vi "Autonomous Independent.vi"() -> ()   [LabVIEW 2016]
doc: "This VI is called when autonomous begins, and will automatically be terminated when autonomous ends. You can carry out timed or sensor driven robot movement independently without needing to return to the caller."
uses:
  <vilib>/Rock Robotics/WPI/ThirdParty/CanMotor/TalonSRX/WPI_CANTalonSRX_APIFeedbackSelect.ctl
  <vilib>/Rock Robotics/WPI/ThirdParty/CanMotor/TalonSRX/WPI_CANTalonSRX_Params.ctl
  <vilib>/Rock Robotics/WPI/ThirdParty/CanMotor/TalonSRX/WPI_CANTalonSRX_APIControlMode.ctl
  <vilib>/Rock Robotics/WPI/Utilities/WPI_GetSetVariantRefNum.vi
  <vilib>/Rock Robotics/Network Tables/NT Read String.vi
  <vilib>/Rock Robotics/Network Tables/NT Write Numeric Array.vi
  <vilib>/Rock Robotics/WPI/RobotDrive/WPI_RobotDriveArcadeDrive_Standard(NoSaturation).vi
  Robot Global Data.vi
panel:
  out "Distance":dbl
  out "Current":dbl
  out "CURRENT":dbl
  out "Distance 5":dbl
  out "Distance 4":dbl
  out "Distance 3":dbl
  out "RIGHT SIDE":dbl
  out "Encoder Position 4":dbl
  out "Encoder Position 3":dbl
  out "Encoder Position":dbl
  out "Encoder Position 2":dbl
  # "Be sure to right-click and choose Data Operations>>Make Current Value default if you want to save the array values with the VI"
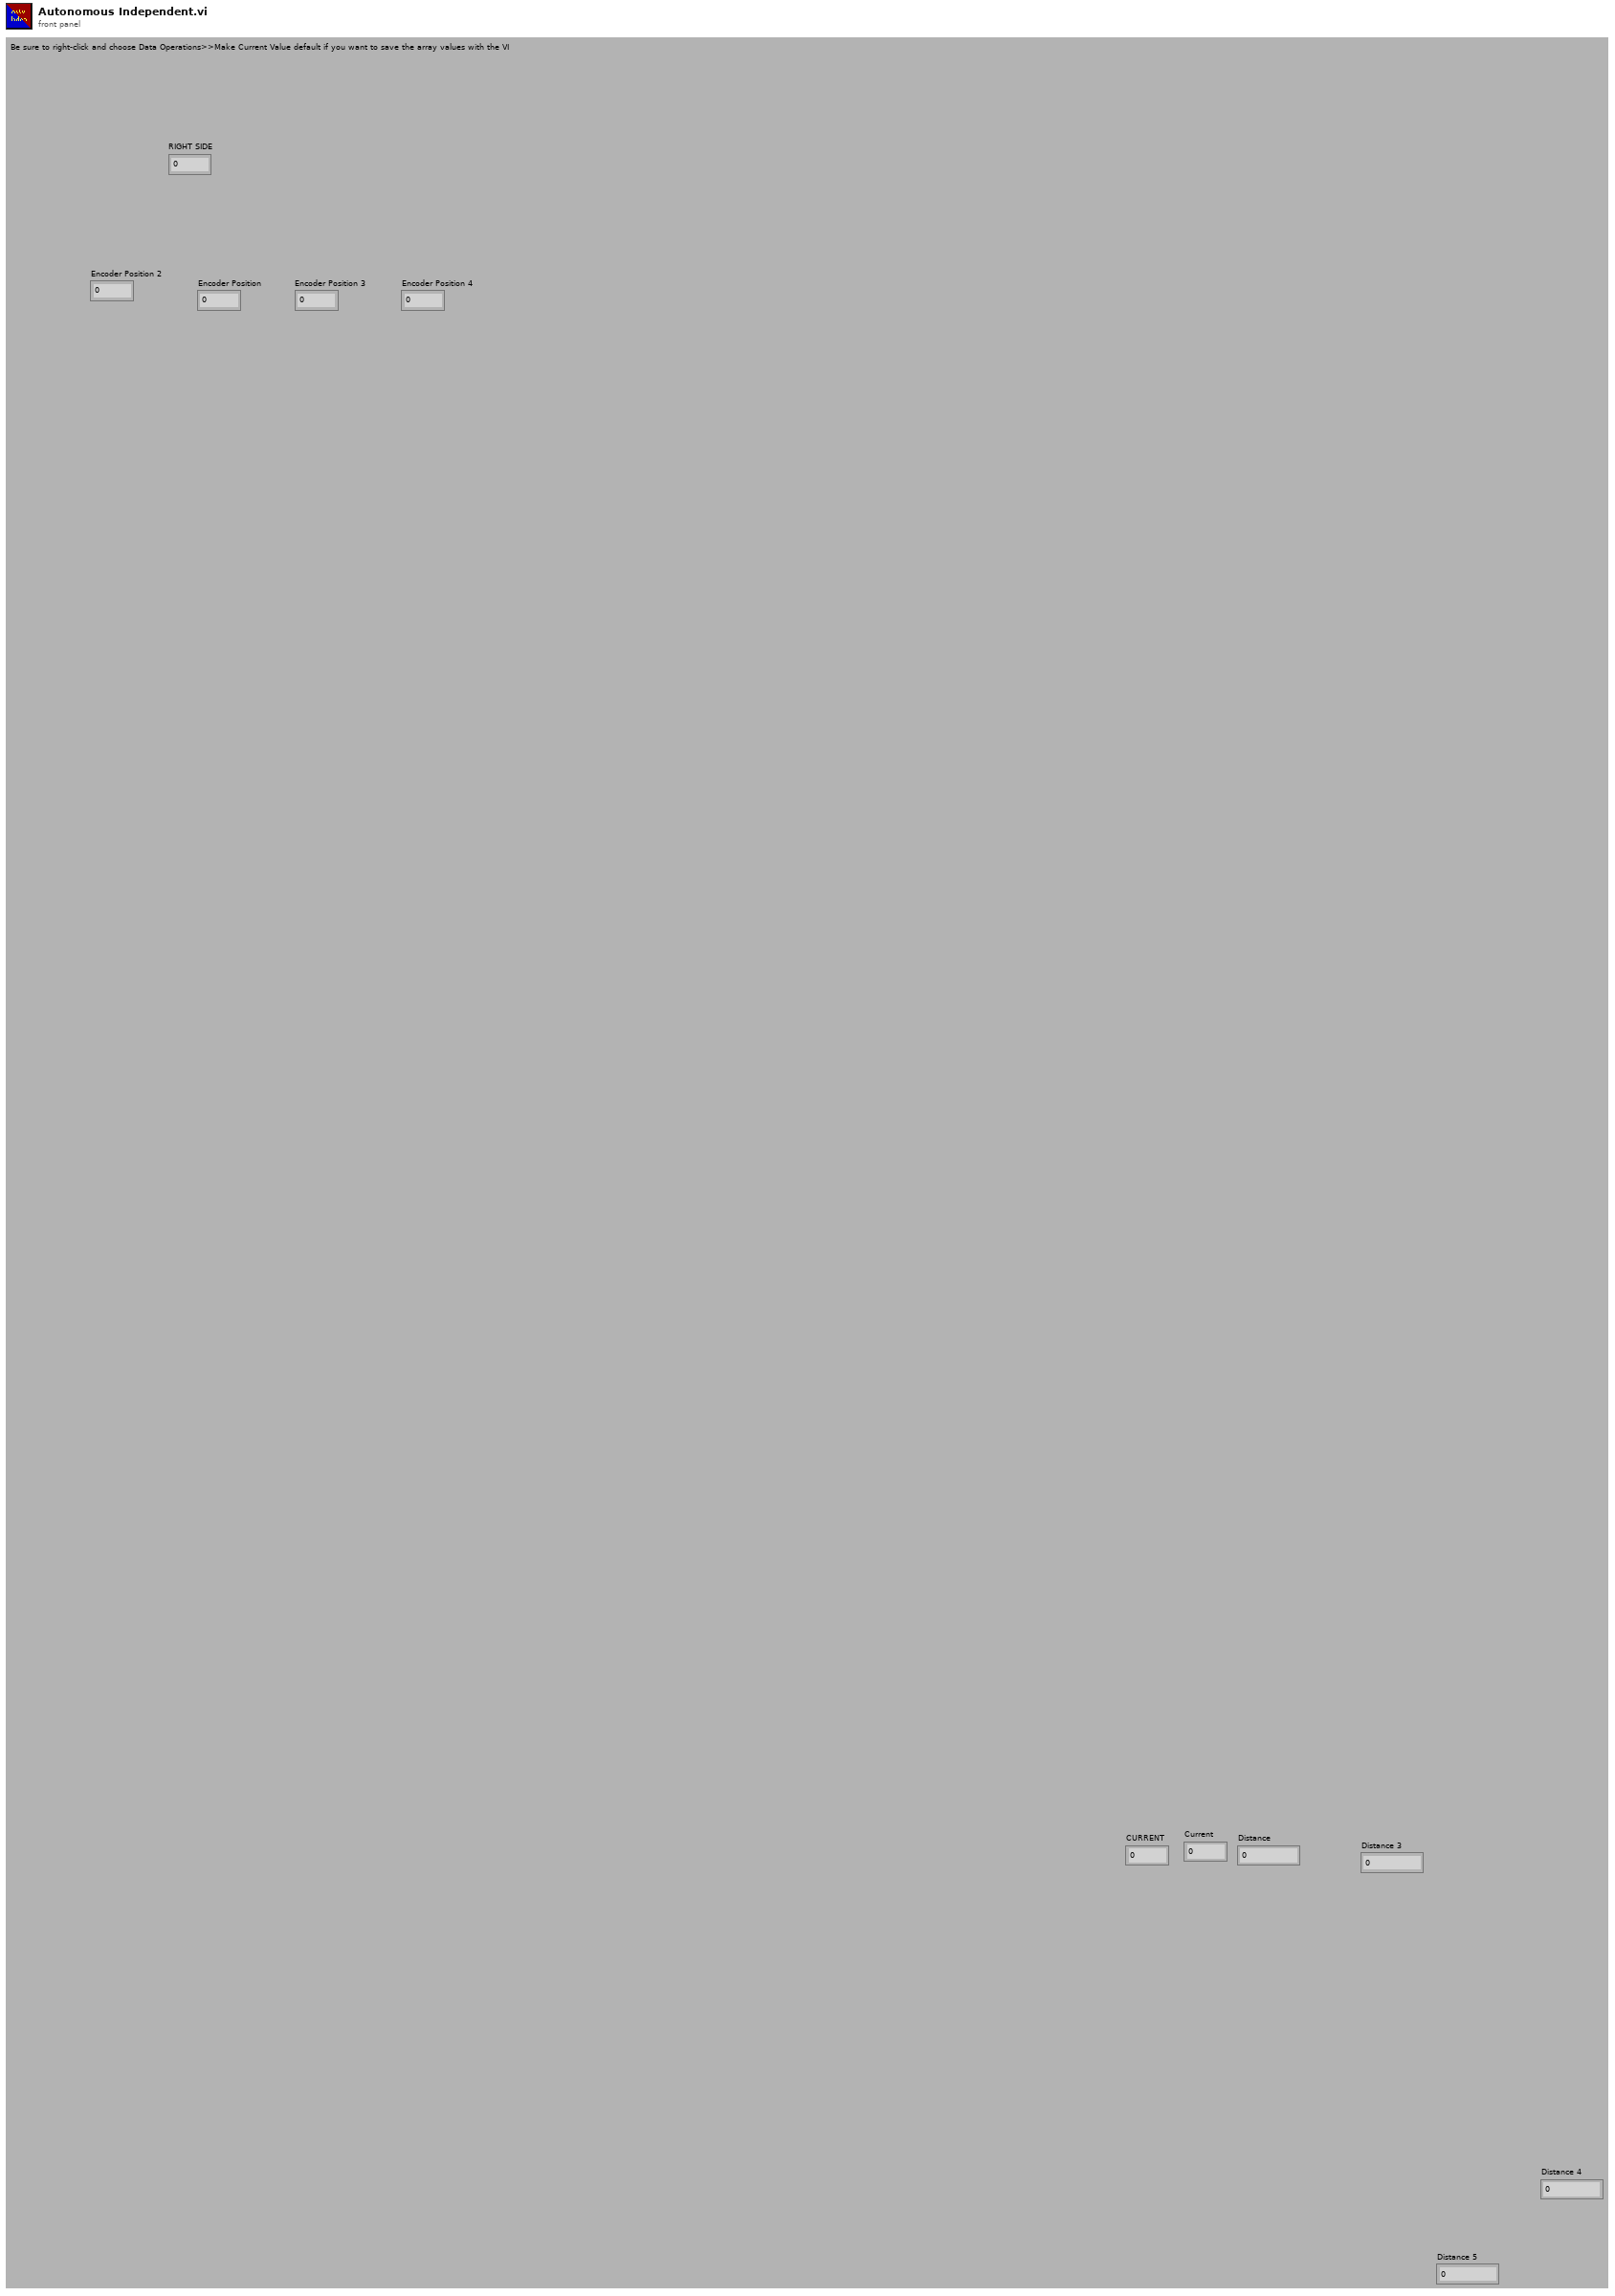
[diagram p1: front panel]
types:
  T1 = typedef "WPI_JoystickDevRef.ctl" = cluster{"Device":T2}
  T2 = typedef "WPI_JoystickDeviceEnum.ctl" = enum16{"USB 0", "USB 1", "USB 2", "USB 3", "USB 4", "USB 5"}
  T3 = typedef "WPI_EncoderDevRef.ctl" = cluster{"DevStatus":errorcluster, "EncoderIndex":T4, "CounterIndex":T5, "DistancePerCount":dbl, "Decoding Type":T6}
  T4 = typedef "FPGA_EncoderIdx.ctl" = enum8{"Enc 0", "Enc 1", "Enc 2", "Enc 3", "Enc 4", "Enc 5", "Enc 6", "Enc 7", "Invalid"}
  T5 = typedef "FPGA_CounterCtrSystemIndex.ctl" = enum8{"Ctr 0", "Ctr 1", "Ctr 2", "Ctr 3", "Ctr 4", "Ctr 5", "Ctr 6", "Ctr 7", "Invalid"}
  T6 = typedef "WPI_EncoderType.ctl" = enum16{"1x", "2x", "4x"}
  T7 = typedef "WPI_MotorControlDeviceRef.ctl" = cluster{"DeviceStatus":errorcluster, "Type":T8, "PWM":cluster{"PWM Channel":T9, "DeadBand":T10}, "CAN":cluster{"Device Number":u8, "SetOutput VI Ref":variant, "GetOutput VI Ref":variant, "Enable VI Ref":variant, "Disable VI Ref":variant, "Data":variant}, "Invert":bool}
  T8 = typedef "WPI_MotorControlType.ctl" = enum16{"PWM", "CAN"}
  T9 = typedef "FPGA_DIOPWMChannel.ctl" = enum8{"PWM 0", "PWM 1", "PWM 2", "PWM 3", "PWM 4", "PWM 5", "PWM 6", "PWM 7", "PWM 8", "PWM 9", "PWM MXP 0", "PWM MXP 1", "PWM MXP 2", "PWM MXP 3", "PWM MXP 4", "PWM MXP 5", "PWM MXP 6", "PWM MXP 7", "PWM MXP 8", "PWM MXP 9", "Invalid"}
  T10 = typedef "WPI_PWMDeadband.ctl" = cluster{"Name":string, "maxPositivePwm":i32, "minPositivePwm":i32, "centerPwm":i32, "maxNegativePwm":i32, "minNegativePwm":i32, "angularRange":u16}
  T11 = typedef "WPI_RobotDriveDevRef.ctl" = cluster{"DevStatus":errorcluster, "Motors[]":T7[], "Square Inputs":bool, "Max Output":dbl}
  T12 = typedef "WPI_CANTalonSRX_APIFeedbackSelect.ctl" = enum16{"Digital Quadrature Encoder", "Analog Potentiometer", "Analog Encoder", "Count on Quad-A (Rising-Edge)", "Count on Quad-A (Falling-Edge)", "CTR Magnetic Enc (Absolute)", "CTR Magnetic Enc (Relative)", "Pulse Width"}
  T13 = typedef "WPI_CANTalonSRX_APIControlMode.ctl" = enum8{"Percent VBus", "Speed", "Position", "Slave", "Unchanged / Invalid", "Voltage Compensation", "Current", "Motion Profile", "Motion Magic"}
  T14 = typedef "WPI_CANTalonSRX_Params.ctl" = u8
  T15 = typedef "WPI_CANTalonSRX_GlobalStatus.ctl" = cluster{"Applied Throttle":dbl, "Module Enabled":bool, "CAN Error":errorcluster, "Closed Loop Error":dbl, "Forward Limit Switch Closed":bool, "Reverse Limit Switch Closed":bool, "Sensor Position":dbl, "Sensor Velocity":dbl, "Current":dbl, "Sticky Fault - Over Temp":bool, "Sticky Fault - Under Voltage":bool, "Sticky Fault - Forward Limit":bool, "Sticky Fault - Reverse Limit":bool, "Sticky Fault - Forward Soft Limit":bool, "Sticky Fault - Reverse Soft Limit":bool, "Brake is Enabled":bool, "Encoder Position":dbl, "Encoder Velocity":dbl, "Encoder Index Count":dbl, "Encoder A Pin State":bool, "Encoder B Pin State":bool, "Encoder Index Pin State":bool, "Analog In":dbl, "Analog In Velocity":dbl, "Temperature (C)":dbl, "Battery Voltage":dbl, "Control 5 Is Supported":bool, "Current Profile Slot Select":dbl, "Pos Div 8":bool, "Vel Div 4":bool, "Pulse Width Position":i32, "Pulse Width Velocity":i32, "Pulse Width Rise To Rise (us)":i32, "Pulse Width Rise To Fall (us)":i32, "Mot Prof Active Is Under Run":bool, "Mot Prof Active Has Under Run":bool, "Mot Prof Active Is Last":bool, "Mot Prof Active Velocity Only":bool, "Mot Prof Active Is Valid":bool, "Mot Prof Buffer Is Full":bool, "Mot Prof Active Profile Slot Select":i32, "Mot Prof NextID":i32, "Mot Prof Count":i32, "Mot Prof Active Velocity":dbl, "Mot Prof Active Position":dbl, "Mot Prof Output Enable":i32, "UsageFrame":u32}
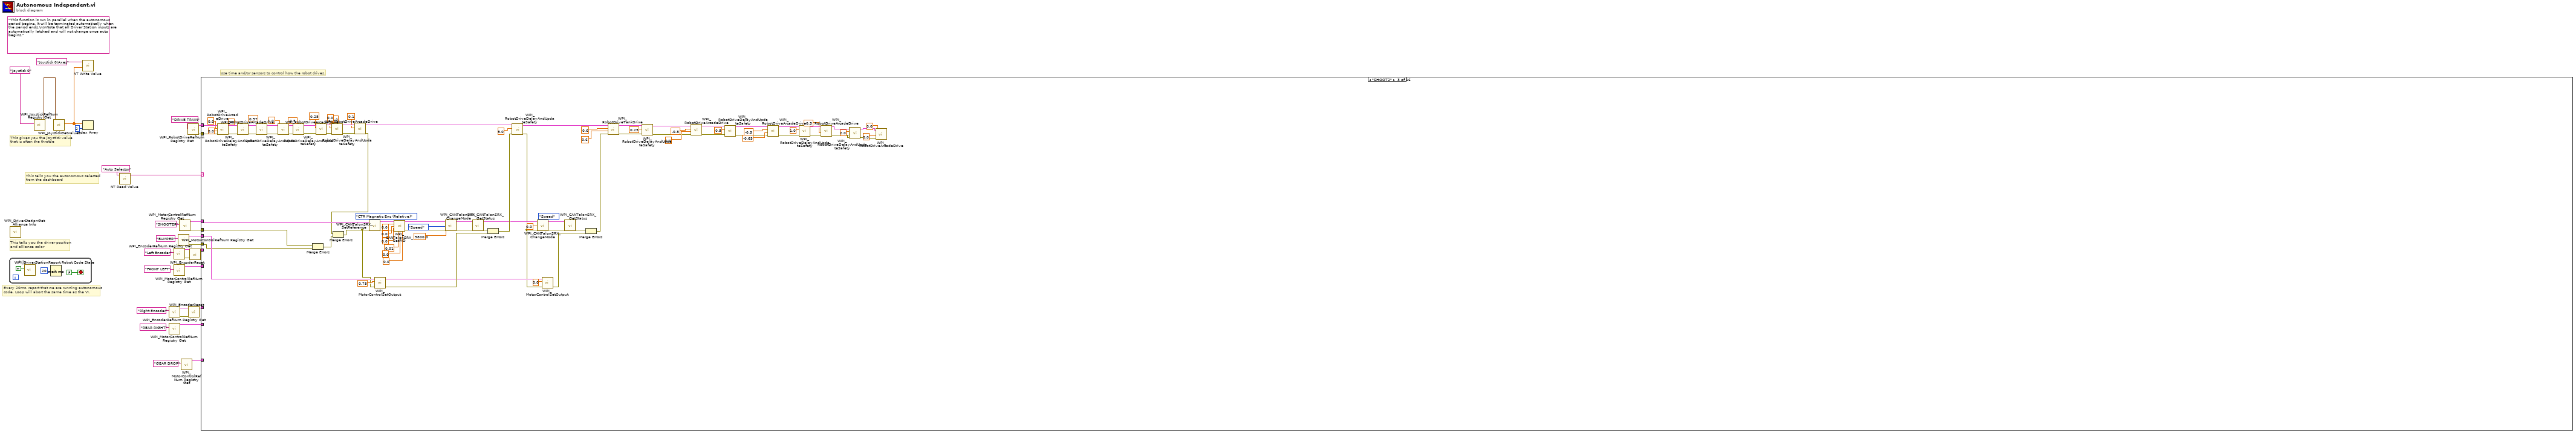
[diagram p0: block diagram]
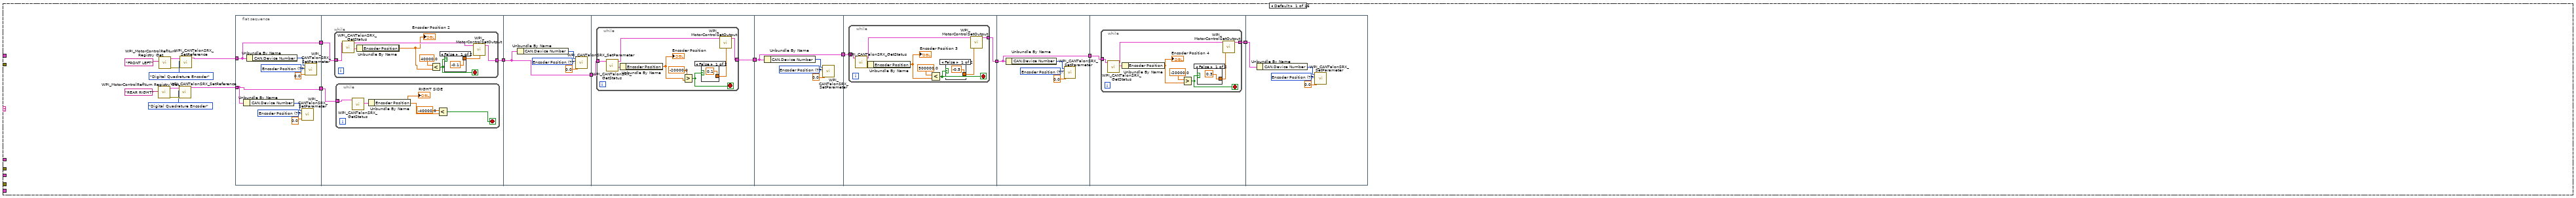
[diagram p2: hidden frame]
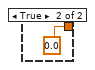
[diagram p3: hidden frame]
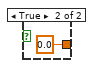
[diagram p4: hidden frame]
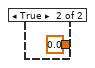
[diagram p5: hidden frame]
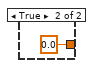
[diagram p6: hidden frame]
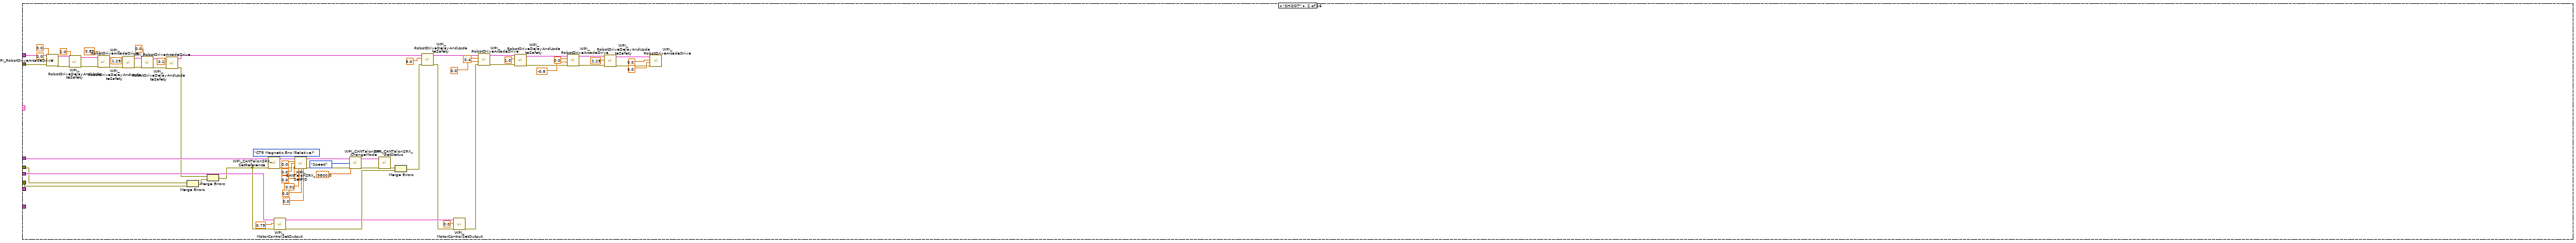
[diagram p7: hidden frame]
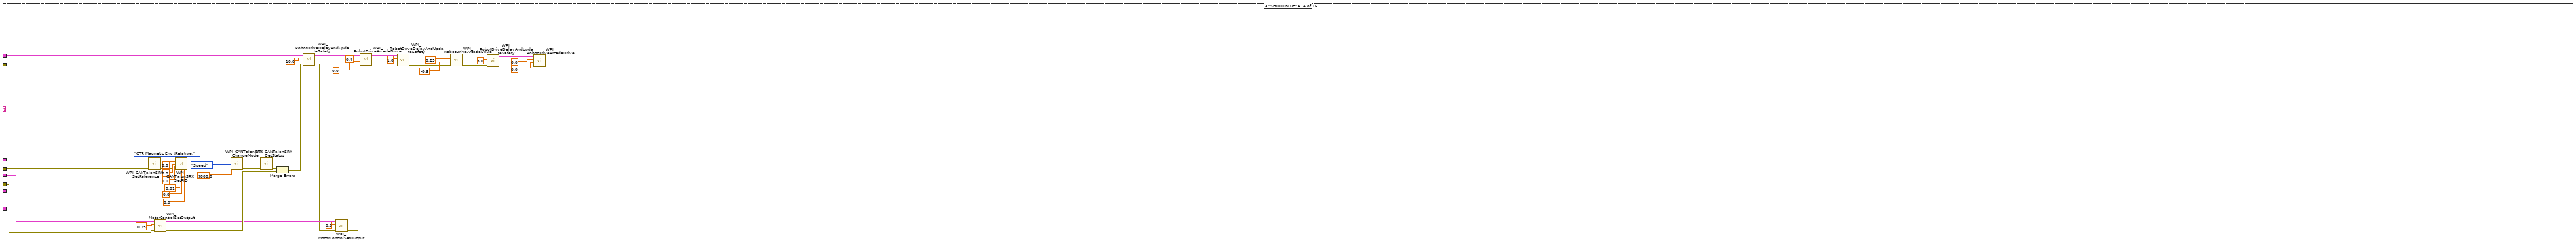
[diagram p8: hidden frame]
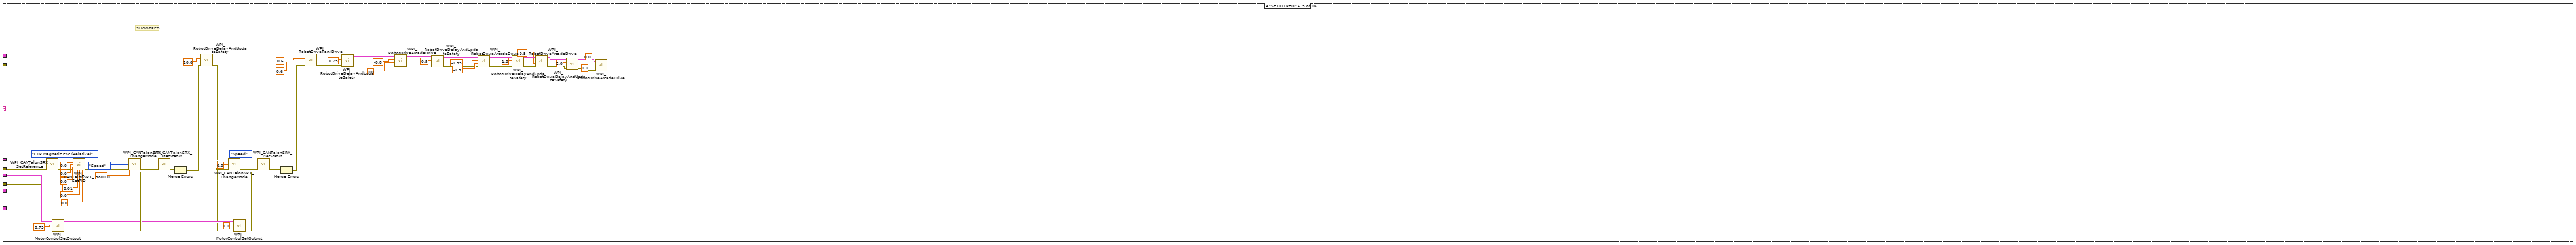
[diagram p9: hidden frame]
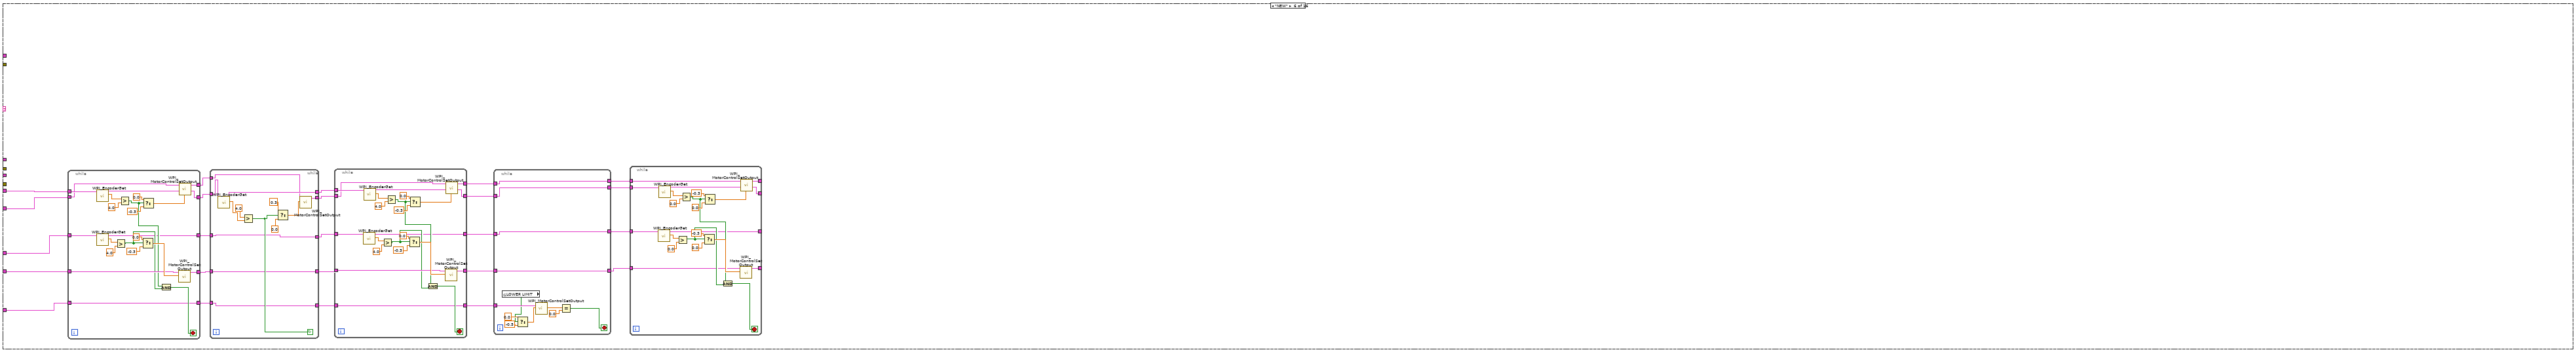
[diagram p10: hidden frame]
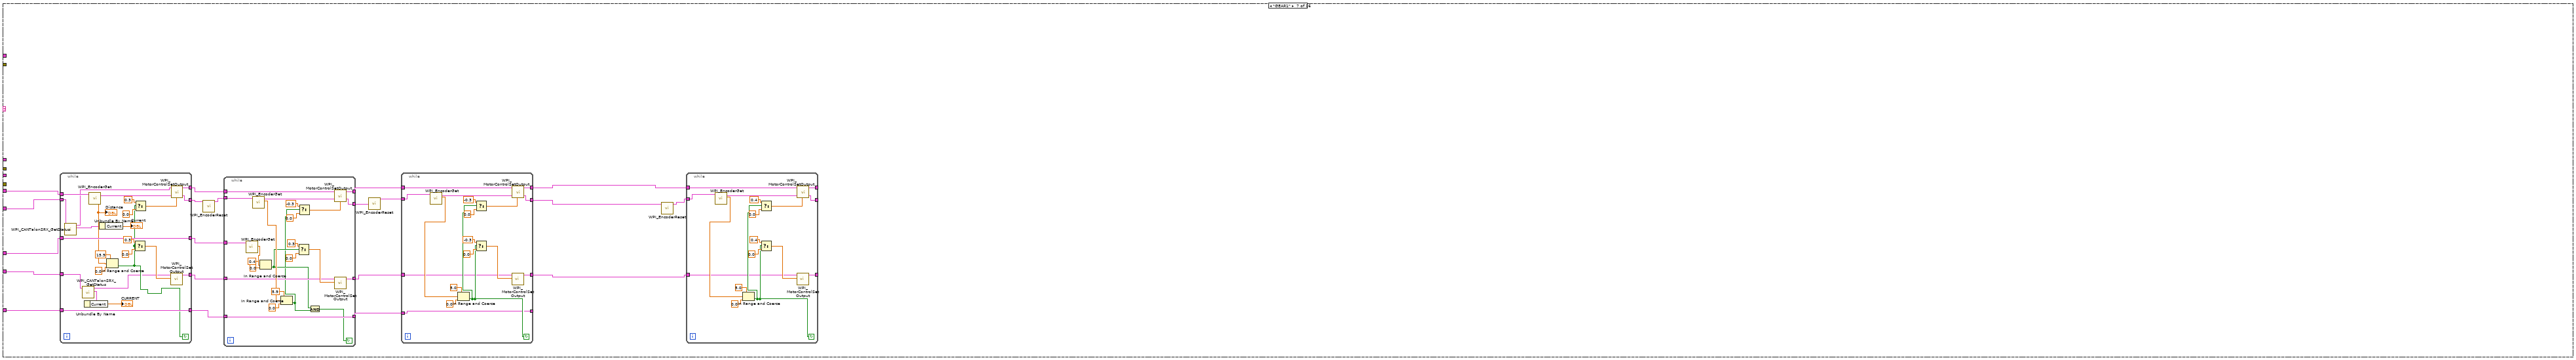
[diagram p11: hidden frame]
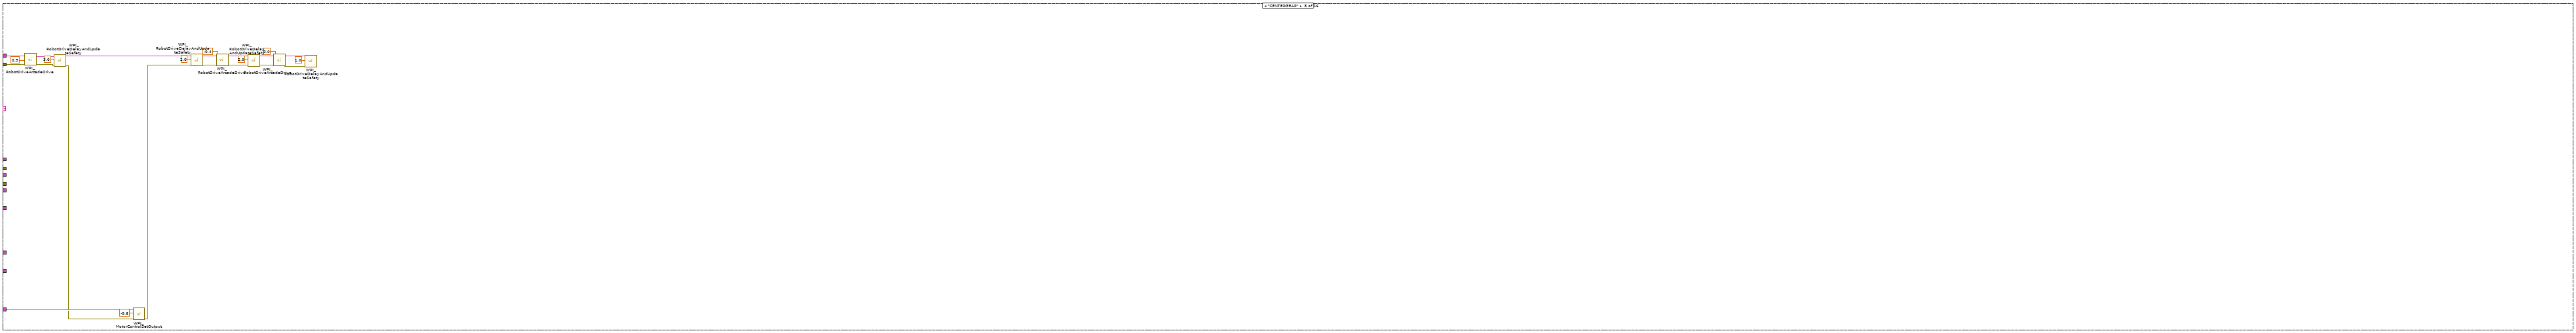
[diagram p12: hidden frame]
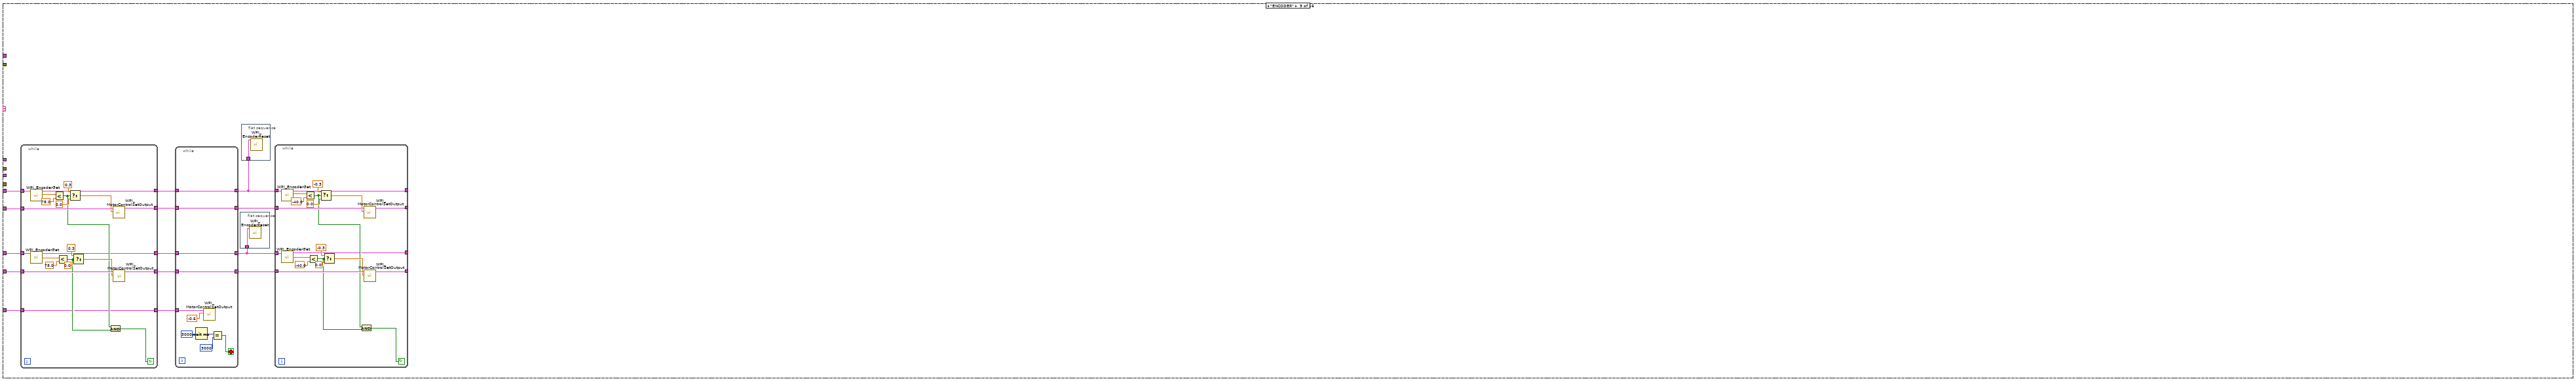
[diagram p13: hidden frame]
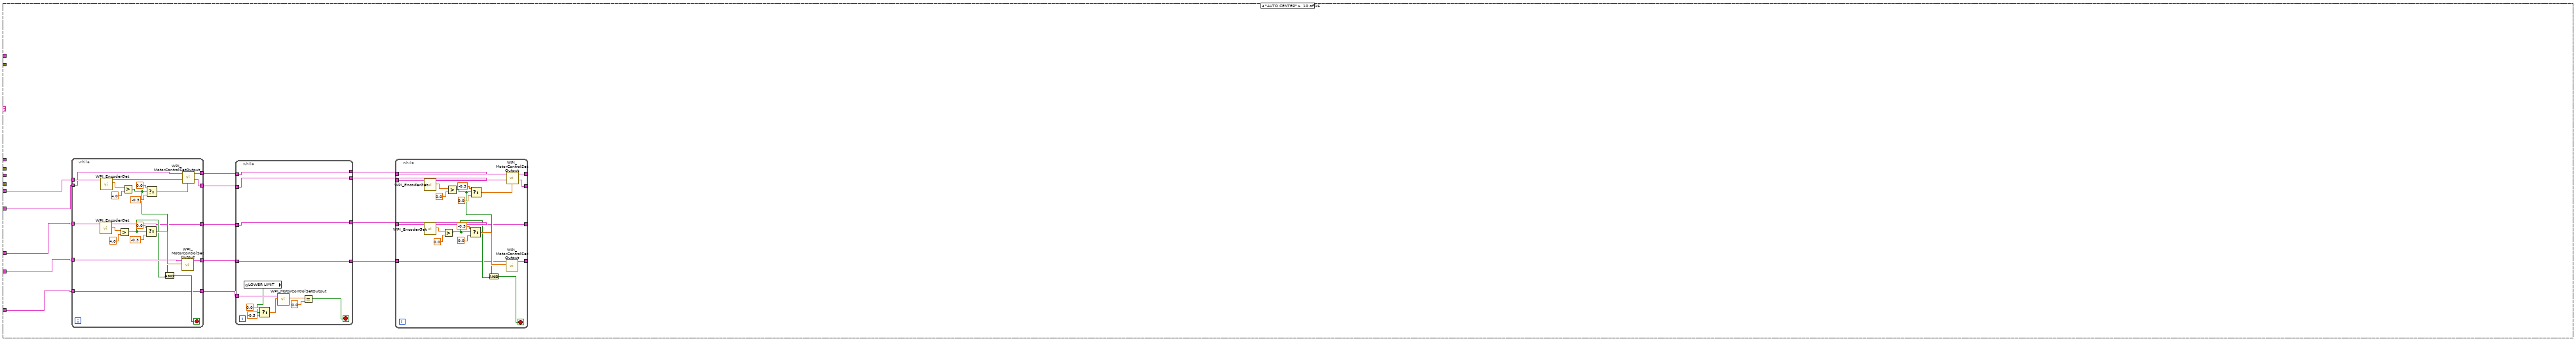
[diagram p14: hidden frame]
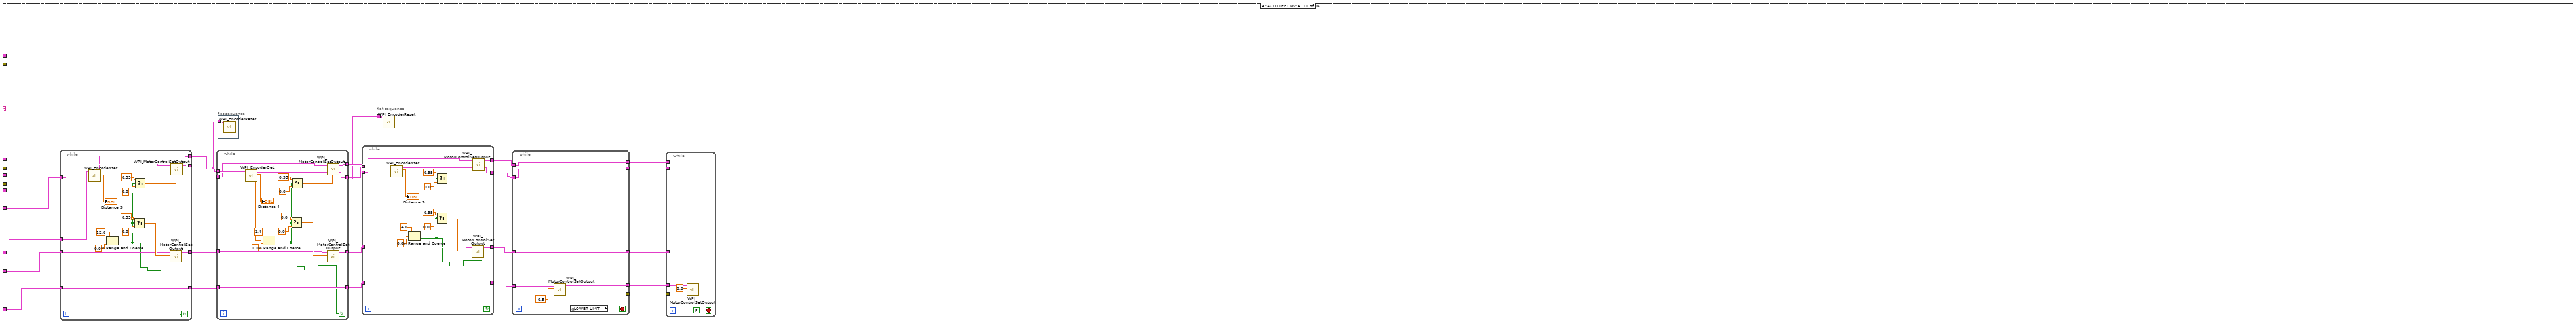
[diagram p15: hidden frame]
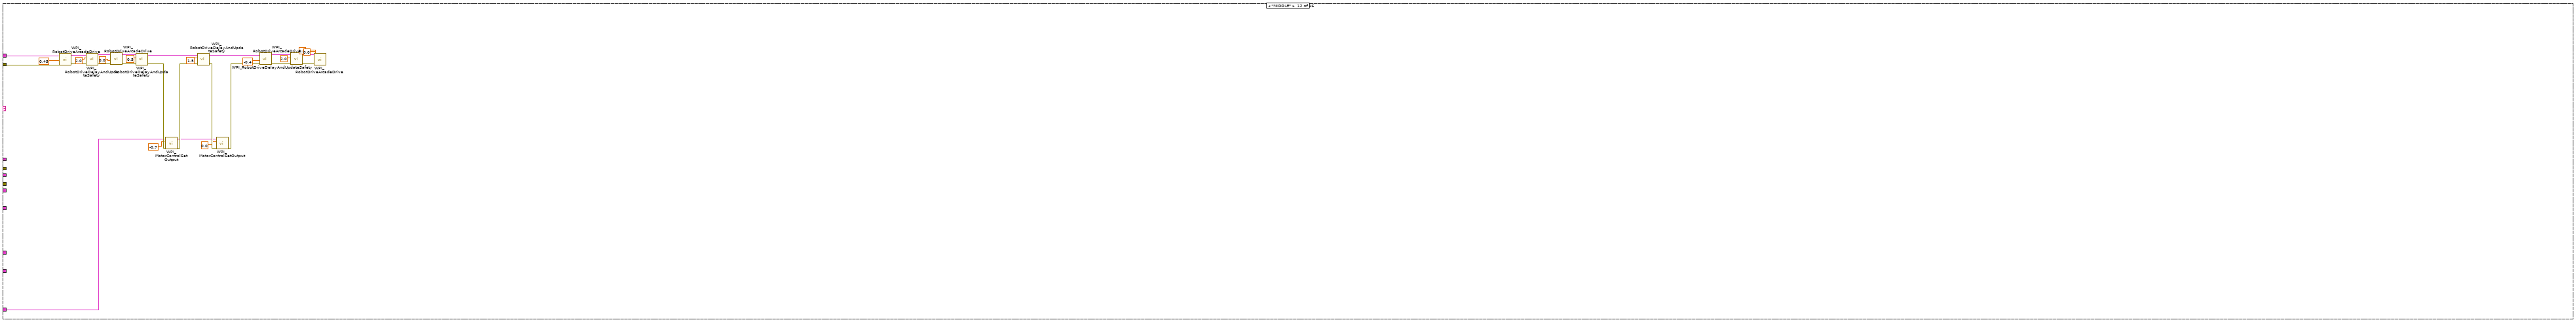
[diagram p16: hidden frame]
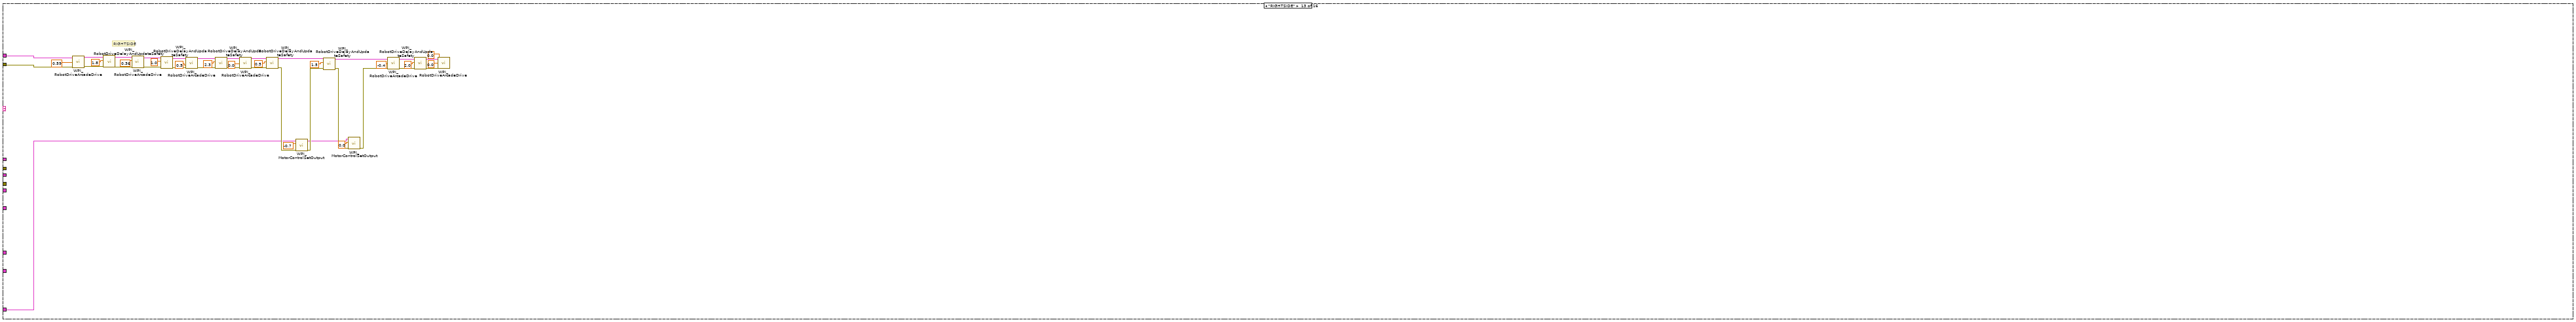
[diagram p17: hidden frame]
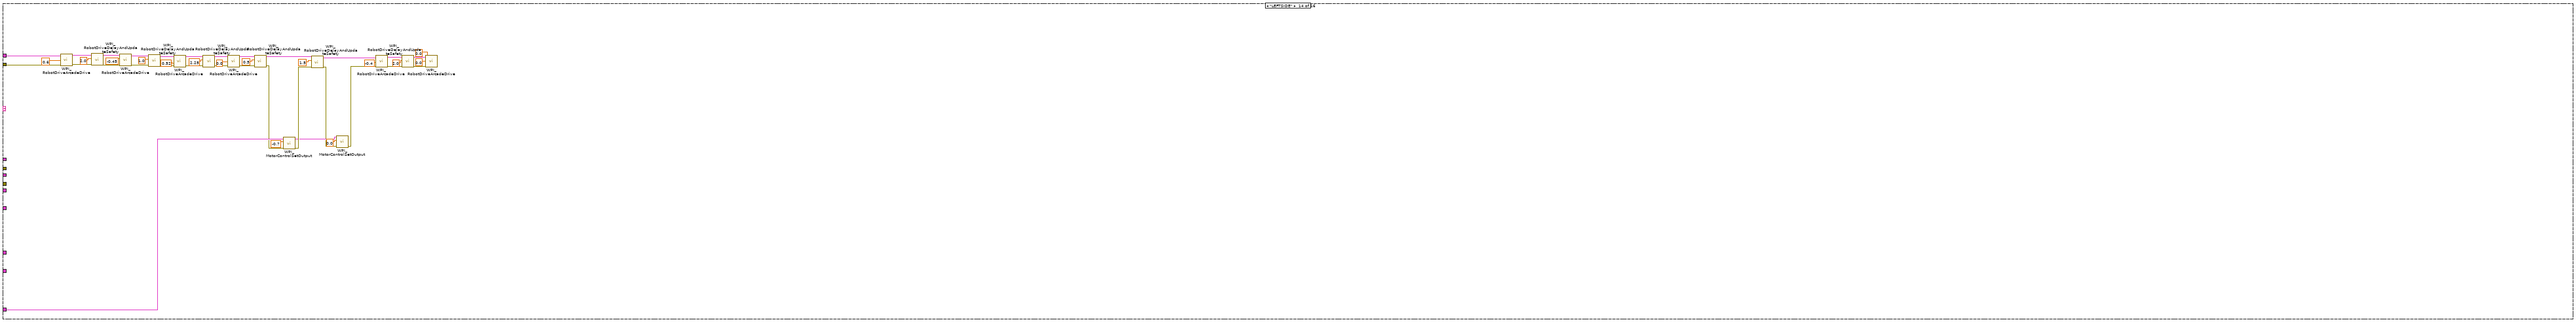
[diagram p18: hidden frame]
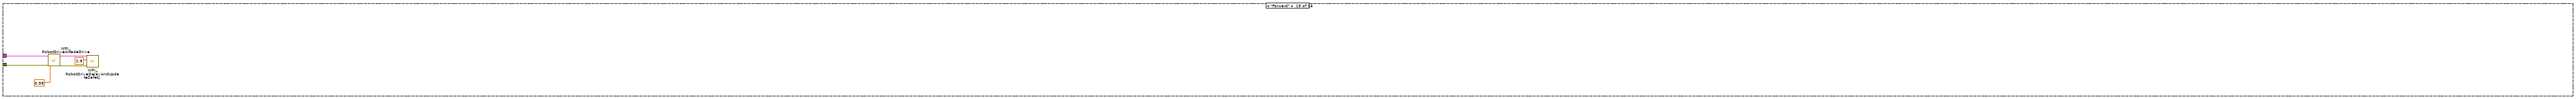
[diagram p19: hidden frame]
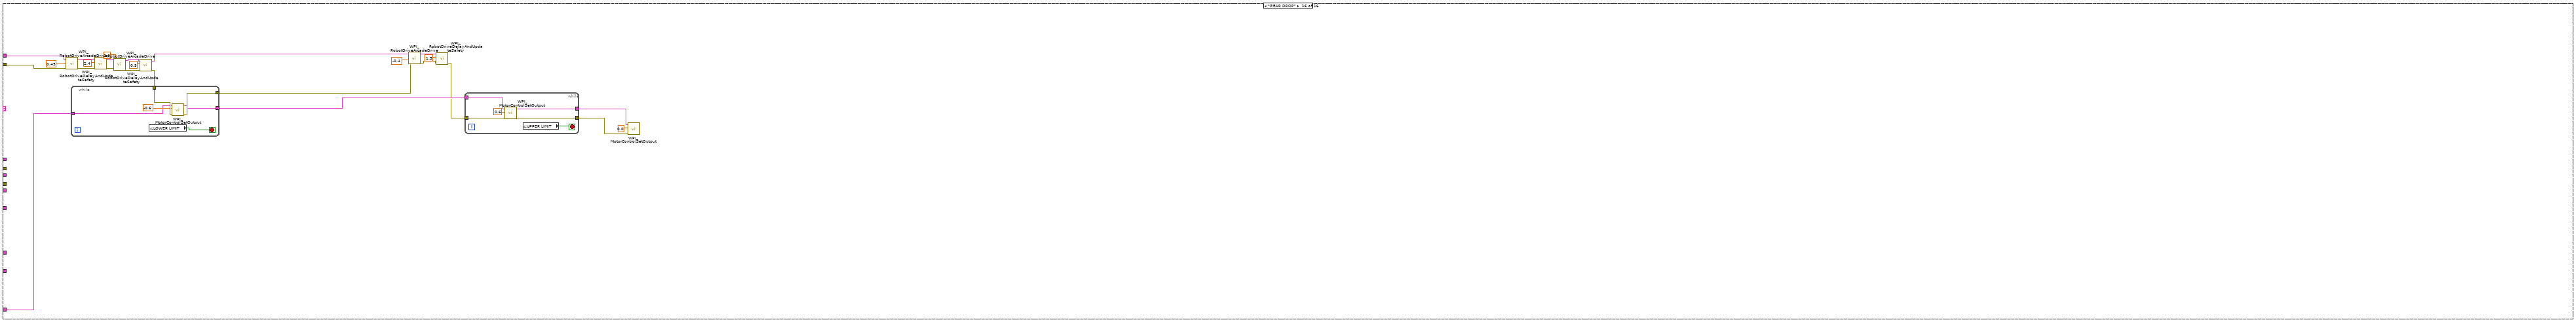
[diagram p20: hidden frame]
diagram:
  (unwired) "This function is run in parallel when the autonomous period begins. It will be terminated automatically when the period ends.\n\nNote that all Driver Station inputs are automatically latched and will not change once auto begins."
  # "Use time and/or sensors to control how the robot drives."
  # "This tells you the autonomous selected\nfrom the dashboard"
  # "Every 20ms, report that we are running autonomous\ncode. Loop will abort the same time as the VI."
  # "This gives you the joystick value\nthat is often the throttle"
  # "This tells you the driver position\nand alliance color"
  n1 = while {
    stop <- FALSE stop-if-true
    n2 = call <vilib>:"WPI_DriverStationReport Robot Code State.vi"("Autonomous"=TRUE) -> ()  [unwired: 10 in, 1 out]
    n3 = Wait (ms)(milliseconds to wait=u32 20) -> ()  [unwired: 1 out]
  }
  n4 = call <vilib>:"WPI_DriverStationGet Alliance Info.vi"() -> ()  [unwired: 12 out]
  n5 = call <vilib>:"WPI_JoystickRefNum Registry Get.vi"("refnum name"="Joystick 0") -> ("JoystickDevRef"=w29:T1)  [unwired: 1 in, 9 out]
  n6 = call <vilib>:"WPI_JoystickGetValues.vi"("JoystickDevRef"=w29) -> ("Axes"=w25:dbl[])  [unwired: 6 in, 4 out]
  n7 = call-poly <vilib>:"NT Write Value.vi"("Numeric Array"=w25, "Name"="Joystick 0/Axes") -> ()  [unwired: 9 in, 1 out]
  n8 = Index Array(array=w25, index=2) -> ()  [unwired: 1 out]
  n9 = call-poly <vilib>:"NT Read Value.vi"("Name"="Auto Selector") -> ("String"=w26:string)  [unwired: 9 in, 1 out]
  n10 = call <vilib>:"WPI_EncoderRefNum Registry Get.vi"("refnum name"="Right Encoder") -> ("error out"=w6:errorcluster, "EncoderDevRef"=w5:T3)  [unwired: 9 in]
  n11 = call <vilib>:"WPI_MotorControlRefNum Registry Get.vi"("refnum name"="REAR RIGHT") -> ("MotorControlDevRef"=w7:T7)  [unwired: 9 in, 1 out]
  n12 = call <vilib>:"WPI_EncoderRefNum Registry Get.vi"("refnum name"="Left Encoder") -> ("error out"=w3:errorcluster, "EncoderDevRef"=w2:T3)  [unwired: 9 in]
  n13 = call <vilib>:"WPI_MotorControlRefNum Registry Get.vi"("refnum name"="FRONT LEFT") -> ("MotorControlDevRef"=w10:T7)  [unwired: 9 in, 1 out]
  n14 = call <vilib>:"WPI_MotorControlRefNum Registry Get.vi"("refnum name"="BUMPER") -> ("error out"=w14:errorcluster, "MotorControlDevRef"=w15:T7)  [unwired: 9 in]
  n15 = call <vilib>:"WPI_MotorControlRefNum Registry Get.vi"("refnum name"="SHOOTER") -> ("error out"=w16:errorcluster, "MotorControlDevRef"=w17:T7)  [unwired: 9 in]
  n16 = call <vilib>:"WPI_MotorControlRefNum Registry Get.vi"("refnum name"="GEAR DROP") -> ("MotorControlDevRef"=w19:T7)  [unwired: 9 in, 1 out]
  n17 = call <vilib>:"WPI_RobotDriveRefNum Registry Get.vi"("refnum name"="DRIVE TRAIN") -> ("error out"=w21:errorcluster, "RobotDriveDevRef"=w22:T11)  [unwired: 9 in]
  n18 = call <vilib>:"WPI_EncoderReset.vi"("error in (no error)"=w6, "EncoderDevRef"=w5) -> ("EncoderDevRef"=w4:T3)  [unwired: 8 in, 1 out]
  n19 = call <vilib>:"WPI_EncoderReset.vi"("error in (no error)"=w3, "EncoderDevRef"=w2) -> ("EncoderDevRef"=w1:T3)  [unwired: 8 in, 1 out]
  n20 = case shown="\"SHOOT2\"" w26 {
    tunnel: w22 -> [_ w156 w231 w298 w387 _ _ w643 _ _ _ w898 w901 w984 w990 w1015]
    tunnel: w21 -> [_ w155 w232 _ _ _ _ w642 _ _ _ w897 w900 w983 w989 w1014]
    tunnel: w19 -> [_ _ _ _ _ w413 w535 w637 w653 w722 w800 w885 w899 w960 _ w995]
    tunnel: w17 -> [_ w186 w214 w294 w393 _ _ _ _ _ _ _ _ _ _ _]
    tunnel: w16 -> [_ w143 w212 w295 w392 _ _ _ _ _ _ _ _ _ _ _]
    tunnel: w15 -> [_ w173 w213 w297 w380 _ _ _ _ _ _ _ _ _ _ _]
    tunnel: w14 -> [_ w142 w211 w296 w379 _ _ _ _ _ _ _ _ _ _ _]
    tunnel: w1 -> [_ _ _ _ _ w427 w538 _ w657 w726 _ _ _ _ _ _]
    tunnel: w10 -> [_ _ _ _ _ w426 w539 _ w656 w725 w802 _ _ _ _ _]
    tunnel: w7 -> [_ _ _ _ _ w424 w536 _ w654 w723 w801 _ _ _ _ _]
    tunnel: w4 -> [_ _ _ _ _ w425 w537 _ w655 w724 w782 _ _ _ _ _]
    frame Default {
      n21 = call <vilib>:"WPI_MotorControlRefNum Registry Get.vi"("refnum name"="REAR RIGHT") -> ("error out"=w38:errorcluster, "MotorControlDevRef"=w37:T7)  [unwired: 9 in]
      n22 = call <vilib>:"WPI_MotorControlRefNum Registry Get.vi"("refnum name"="FRONT LEFT") -> ("error out"=w50:errorcluster, "MotorControlDevRef"=w51:T7)  [unwired: 9 in]
      n23 = call <vilib>:"WPI_CANTalonSRX_SetReference.vi"("error in (no error)"=w38, "Feedback Reference"=WPI_CANTalonSRX_APIFeedbackSelect."Digital Quadrature Encoder", "CAN Talon SRX Ref"=w37) -> ("CAN Talon SRX Ref"=w35:T7)  [unwired: 7 in, 1 out]
      n24 = call <vilib>:"WPI_CANTalonSRX_SetReference.vi"("error in (no error)"=w50, "Feedback Reference"=WPI_CANTalonSRX_APIFeedbackSelect."Digital Quadrature Encoder", "CAN Talon SRX Ref"=w51) -> ("CAN Talon SRX Ref"=w46:T7)  [unwired: 7 in, 1 out]
      n25 = flat-sequence {
        tunnel: w46 -> [w57]
        tunnel: [w57] -> w45
        tunnel: w35 -> [w53]
        tunnel: [w53] -> w34
        tunnel: [w62] -> w48
        tunnel: w45 -> [w63]
        tunnel: w34 -> [w61]
        tunnel: w48 -> [w79]
        tunnel: [w79] -> w47
        tunnel: w47 -> [w84]
        tunnel: [w83] -> w44
        tunnel: w44 -> [w95]
        tunnel: [w95] -> w43
        tunnel: w43 -> [w100]
        tunnel: [w99] -> w42
        tunnel: w42 -> [w111]
        tunnel: [w111] -> w41
        tunnel: w41 -> [w116]
        tunnel: [w115] -> w40
        tunnel: w40 -> [w127]
        frame #0 {
          w55 = T14 77 items=["Slot 0 - P"=1, "Slot 0 - I"=2, "Slot 0 - D"=3, "Slot 0 - F"=4, "Slot 0 - I Zone"=5, "Slot 0 - Ramp Rate"=6, "Slot 1 - P"=11, "Slot 1 - I"=12, "Slot 1 - D"=13, "Slot 1 - F"=14, "Slot 1 - I Zone"=15, "Slot 1 - Ramp Rate"=16, "Soft Limit - Forward"=21, "Soft Limit - Reverse"=22, "Soft Limit - Forward Enable"=23, "Soft Limit - Reverse Enable"=24, "On Boot - Brake Mode"=31, "On Boot - Limit Normally Closed - Forward"=32, "On Boot - Limit Normally Closed - Reverse"=33, "On Boot - Limit Disabled - Forward"=34, "On Boot - Limit Disabled - Reverse"=35, "Fault - Over Temp"=41, "Fault - Under Voltage"=42, "Fault - Forward Limit"=43, "Fault - Reverse Limit"=44, "Fault - Hardware Failure"=45, "Fault - Forward Soft Limit"=46, "Fault - Reverse Soft Limit"=47, "Sticky Fault - Over Temp"=48, "Sticky Fault - Under Voltage"=49, "Sticky Fault - Forward Limit"=50, "Sticky Fault - Reverse Limit"=51, "Sticky Fault - Forward Soft Limit"=52, "Sticky Fault - Reverse Soft Limit"=53, "Applied Throttle"=61, "Closed-Loop Error"=62, "Select Feedback Device"=63, "Reverse Closed-Loop Output"=64, "Mode Select"=65, "Profile Slot Select"=66, "Ramp Throttle"=67, "Reverse Feedback Sensor"=68, "Limit Switch Enabled"=69, "Limit Switch Closed - Forward"=70, "Limit Switch Closed - Reverse"=71, "Sensor Position"=73, "Sensor Velocity"=74, "Current"=75, "Brake is Enabled"=76, "Encoder Position"=77, "Encoder Velocity"=78, "Encoder Index Rise Events"=79, "Encoder A Pin State"=80, "Encoder B Pin State"=81, "Encoder Index Pin State"=82, "Analog In with Overflow"=83, "Analog In Velocity"=84, "Temperature"=85, "Battery Voltage"=86, "Reset Count"=87, "Reset Flags"=88, "Firmware Version"=89, "Settings Changed"=90, "Quad Filter Enable"=91, "Ignore Disable Broadcast"=92, "I Accumulator"=93, "Status 1 Frame Rate Ms"=94, "Status 2 Frame Rate Ms"=95, "Status 3 Frame Rate Ms"=96, "Status 4 Frame Rate Ms"=97, "Status 6 Frame Rate Ms"=98, "Status 7 Frame Rate Ms"=99, "Enable Index Pin Clear Position"=100, "Peak Positive Output"=104, "Nominal Positive Output"=105, "Peak Negative Output"=106, "Nominal Negative Output"=107, "Quad Index Pin Polarity"=108, "Status 8 Frame Rate Ms"=109, "Allow Position Overflow"=110, "Slot 0 - Allowable Closed-Loop Error"=111, "Number Potentiometer Turns"=112, "Encoder Codes Per Rev"=113, "Pulse Width Decoded Position"=114, "Analog Position"=115, "Voltage Compensation Rate (V/s)"=116, "Slot 1 - Allowable Closed-Loop Error"=117, "Motion Profile Has Underrun Err"=119, "Reserved 120"=120, "Legacy Control Mode"=121, "Motion Magic Acceleration"=122, "Motion Magic Cruise Velocity"=123, "Status 10 Frame Rate"=124, "Current Limit Threshold"=125, "CustomParam0"=137, "CustomParam1"=138, "PersStorageSaving"=139, "ClearPositionOnLimitF"=144, "ClearPositionOnLimitR"=145, "NominalBatteryVoltage"=146, "SampleVelocityPeriod"=147, "SampleVelocityWindow"=148] ("Parameter")
          w59 = T14 77 items=["Slot 0 - P"=1, "Slot 0 - I"=2, "Slot 0 - D"=3, "Slot 0 - F"=4, "Slot 0 - I Zone"=5, "Slot 0 - Ramp Rate"=6, "Slot 1 - P"=11, "Slot 1 - I"=12, "Slot 1 - D"=13, "Slot 1 - F"=14, "Slot 1 - I Zone"=15, "Slot 1 - Ramp Rate"=16, "Soft Limit - Forward"=21, "Soft Limit - Reverse"=22, "Soft Limit - Forward Enable"=23, "Soft Limit - Reverse Enable"=24, "On Boot - Brake Mode"=31, "On Boot - Limit Normally Closed - Forward"=32, "On Boot - Limit Normally Closed - Reverse"=33, "On Boot - Limit Disabled - Forward"=34, "On Boot - Limit Disabled - Reverse"=35, "Fault - Over Temp"=41, "Fault - Under Voltage"=42, "Fault - Forward Limit"=43, "Fault - Reverse Limit"=44, "Fault - Hardware Failure"=45, "Fault - Forward Soft Limit"=46, "Fault - Reverse Soft Limit"=47, "Sticky Fault - Over Temp"=48, "Sticky Fault - Under Voltage"=49, "Sticky Fault - Forward Limit"=50, "Sticky Fault - Reverse Limit"=51, "Sticky Fault - Forward Soft Limit"=52, "Sticky Fault - Reverse Soft Limit"=53, "Applied Throttle"=61, "Closed-Loop Error"=62, "Select Feedback Device"=63, "Reverse Closed-Loop Output"=64, "Mode Select"=65, "Profile Slot Select"=66, "Ramp Throttle"=67, "Reverse Feedback Sensor"=68, "Limit Switch Enabled"=69, "Limit Switch Closed - Forward"=70, "Limit Switch Closed - Reverse"=71, "Sensor Position"=73, "Sensor Velocity"=74, "Current"=75, "Brake is Enabled"=76, "Encoder Position"=77, "Encoder Velocity"=78, "Encoder Index Rise Events"=79, "Encoder A Pin State"=80, "Encoder B Pin State"=81, "Encoder Index Pin State"=82, "Analog In with Overflow"=83, "Analog In Velocity"=84, "Temperature"=85, "Battery Voltage"=86, "Reset Count"=87, "Reset Flags"=88, "Firmware Version"=89, "Settings Changed"=90, "Quad Filter Enable"=91, "Ignore Disable Broadcast"=92, "I Accumulator"=93, "Status 1 Frame Rate Ms"=94, "Status 2 Frame Rate Ms"=95, "Status 3 Frame Rate Ms"=96, "Status 4 Frame Rate Ms"=97, "Status 6 Frame Rate Ms"=98, "Status 7 Frame Rate Ms"=99, "Enable Index Pin Clear Position"=100, "Peak Positive Output"=104, "Nominal Positive Output"=105, "Peak Negative Output"=106, "Nominal Negative Output"=107, "Quad Index Pin Polarity"=108, "Status 8 Frame Rate Ms"=109, "Allow Position Overflow"=110, "Slot 0 - Allowable Closed-Loop Error"=111, "Number Potentiometer Turns"=112, "Encoder Codes Per Rev"=113, "Pulse Width Decoded Position"=114, "Analog Position"=115, "Voltage Compensation Rate (V/s)"=116, "Slot 1 - Allowable Closed-Loop Error"=117, "Motion Profile Has Underrun Err"=119, "Reserved 120"=120, "Legacy Control Mode"=121, "Motion Magic Acceleration"=122, "Motion Magic Cruise Velocity"=123, "Status 10 Frame Rate"=124, "Current Limit Threshold"=125, "CustomParam0"=137, "CustomParam1"=138, "PersStorageSaving"=139, "ClearPositionOnLimitF"=144, "ClearPositionOnLimitR"=145, "NominalBatteryVoltage"=146, "SampleVelocityPeriod"=147, "SampleVelocityWindow"=148] ("Parameter")
          n26 = Unbundle By Name(w53) -> ("CAN.Device Number"=w54:u8)
          n27 = Unbundle By Name(w57) -> ("CAN.Device Number"=w60:u8)
          n28 = call <vilib>:"WPI_CANTalonSRX_SetParameter.vi"("Value"=0.0, "Parameter"=w55, "Device ID (0)"=w54) -> ()  [unwired: 7 in, 2 out]
          n29 = call <vilib>:"WPI_CANTalonSRX_SetParameter.vi"("Value"=0.0, "Parameter"=w59, "Device ID (0)"=w60) -> ()  [unwired: 7 in, 2 out]
        }
        frame #1 {
          n30 = while {
            tunnel: w63 -> [w70]
            tunnel: [w69] -> w62
            stop <- w73 stop-if-true
            n31 = call <vilib>:"WPI_CANTalonSRX_GetStatus.vi"("CAN Talon SRX Ref"=w70) -> ("Talon SRX Status"=w76:T15, "CAN Talon SRX Ref"=w75:T7)  [unwired: 8 in, 1 out]
            n32 = Unbundle By Name(w76) -> ("Encoder Position"=w72:dbl)
            "Encoder Position 2" <- w72
            n33 = Less?(x=40000.0, y=w72) -> (x < y?=w73:bool)
            n34 = case shown="False" w73 {
              tunnel: [-0.1 ("x") 0.0 ("x")] -> w74
              frame False {
              }
              frame True {
              }
            }
            n35 = call <vilib>:"WPI_MotorControlSetOutput.vi"("Output"=w74, "MotorControlDevRef"=w75) -> ("MotorControlDevRef"=w69:T7)  [unwired: 7 in, 2 out]
          }
          n36 = while {
            tunnel: w61 -> [w68]
            stop <- w65 stop-if-true
            n37 = call <vilib>:"WPI_CANTalonSRX_GetStatus.vi"("CAN Talon SRX Ref"=w68) -> ("Talon SRX Status"=w64:T15)  [unwired: 8 in, 2 out]
            n38 = Unbundle By Name(w64) -> ("Encoder Position"=w67:dbl)
            "RIGHT SIDE" <- w67
            n39 = Less?(x=-40000.0, y=w67) -> (x < y?=w65:bool)
          }
        }
        frame #2 {
          w81 = T14 77 items=["Slot 0 - P"=1, "Slot 0 - I"=2, "Slot 0 - D"=3, "Slot 0 - F"=4, "Slot 0 - I Zone"=5, "Slot 0 - Ramp Rate"=6, "Slot 1 - P"=11, "Slot 1 - I"=12, "Slot 1 - D"=13, "Slot 1 - F"=14, "Slot 1 - I Zone"=15, "Slot 1 - Ramp Rate"=16, "Soft Limit - Forward"=21, "Soft Limit - Reverse"=22, "Soft Limit - Forward Enable"=23, "Soft Limit - Reverse Enable"=24, "On Boot - Brake Mode"=31, "On Boot - Limit Normally Closed - Forward"=32, "On Boot - Limit Normally Closed - Reverse"=33, "On Boot - Limit Disabled - Forward"=34, "On Boot - Limit Disabled - Reverse"=35, "Fault - Over Temp"=41, "Fault - Under Voltage"=42, "Fault - Forward Limit"=43, "Fault - Reverse Limit"=44, "Fault - Hardware Failure"=45, "Fault - Forward Soft Limit"=46, "Fault - Reverse Soft Limit"=47, "Sticky Fault - Over Temp"=48, "Sticky Fault - Under Voltage"=49, "Sticky Fault - Forward Limit"=50, "Sticky Fault - Reverse Limit"=51, "Sticky Fault - Forward Soft Limit"=52, "Sticky Fault - Reverse Soft Limit"=53, "Applied Throttle"=61, "Closed-Loop Error"=62, "Select Feedback Device"=63, "Reverse Closed-Loop Output"=64, "Mode Select"=65, "Profile Slot Select"=66, "Ramp Throttle"=67, "Reverse Feedback Sensor"=68, "Limit Switch Enabled"=69, "Limit Switch Closed - Forward"=70, "Limit Switch Closed - Reverse"=71, "Sensor Position"=73, "Sensor Velocity"=74, "Current"=75, "Brake is Enabled"=76, "Encoder Position"=77, "Encoder Velocity"=78, "Encoder Index Rise Events"=79, "Encoder A Pin State"=80, "Encoder B Pin State"=81, "Encoder Index Pin State"=82, "Analog In with Overflow"=83, "Analog In Velocity"=84, "Temperature"=85, "Battery Voltage"=86, "Reset Count"=87, "Reset Flags"=88, "Firmware Version"=89, "Settings Changed"=90, "Quad Filter Enable"=91, "Ignore Disable Broadcast"=92, "I Accumulator"=93, "Status 1 Frame Rate Ms"=94, "Status 2 Frame Rate Ms"=95, "Status 3 Frame Rate Ms"=96, "Status 4 Frame Rate Ms"=97, "Status 6 Frame Rate Ms"=98, "Status 7 Frame Rate Ms"=99, "Enable Index Pin Clear Position"=100, "Peak Positive Output"=104, "Nominal Positive Output"=105, "Peak Negative Output"=106, "Nominal Negative Output"=107, "Quad Index Pin Polarity"=108, "Status 8 Frame Rate Ms"=109, "Allow Position Overflow"=110, "Slot 0 - Allowable Closed-Loop Error"=111, "Number Potentiometer Turns"=112, "Encoder Codes Per Rev"=113, "Pulse Width Decoded Position"=114, "Analog Position"=115, "Voltage Compensation Rate (V/s)"=116, "Slot 1 - Allowable Closed-Loop Error"=117, "Motion Profile Has Underrun Err"=119, "Reserved 120"=120, "Legacy Control Mode"=121, "Motion Magic Acceleration"=122, "Motion Magic Cruise Velocity"=123, "Status 10 Frame Rate"=124, "Current Limit Threshold"=125, "CustomParam0"=137, "CustomParam1"=138, "PersStorageSaving"=139, "ClearPositionOnLimitF"=144, "ClearPositionOnLimitR"=145, "NominalBatteryVoltage"=146, "SampleVelocityPeriod"=147, "SampleVelocityWindow"=148] ("Parameter")
          n40 = Unbundle By Name(w79) -> ("CAN.Device Number"=w82:u8)
          n41 = call <vilib>:"WPI_CANTalonSRX_SetParameter.vi"("Value"=0.0, "Parameter"=w81, "Device ID (0)"=w82) -> ()  [unwired: 7 in, 2 out]
        }
        frame #3 {
          n42 = while {
            tunnel: w84 -> [w86]
            tunnel: [w85] -> w83
            stop <- w89 stop-if-true
            n43 = call <vilib>:"WPI_CANTalonSRX_GetStatus.vi"("CAN Talon SRX Ref"=w86) -> ("Talon SRX Status"=w92:T15, "CAN Talon SRX Ref"=w91:T7)  [unwired: 8 in, 1 out]
            n44 = Unbundle By Name(w92) -> ("Encoder Position"=w88:dbl)
            "Encoder Position" <- w88
            n45 = Greater?(x=-20000.0 ("y"), y=w88) -> (0:w89:bool)
            n46 = case shown="False" w89 {
              tunnel: [0.1 ("x") 0.0 ("x")] -> w90
              frame False {
              }
              frame True {
              }
            }
            n47 = call <vilib>:"WPI_MotorControlSetOutput.vi"("Output"=w90, "MotorControlDevRef"=w91) -> ("MotorControlDevRef"=w85:T7)  [unwired: 7 in, 2 out]
          }
        }
        frame #4 {
          w97 = T14 77 items=["Slot 0 - P"=1, "Slot 0 - I"=2, "Slot 0 - D"=3, "Slot 0 - F"=4, "Slot 0 - I Zone"=5, "Slot 0 - Ramp Rate"=6, "Slot 1 - P"=11, "Slot 1 - I"=12, "Slot 1 - D"=13, "Slot 1 - F"=14, "Slot 1 - I Zone"=15, "Slot 1 - Ramp Rate"=16, "Soft Limit - Forward"=21, "Soft Limit - Reverse"=22, "Soft Limit - Forward Enable"=23, "Soft Limit - Reverse Enable"=24, "On Boot - Brake Mode"=31, "On Boot - Limit Normally Closed - Forward"=32, "On Boot - Limit Normally Closed - Reverse"=33, "On Boot - Limit Disabled - Forward"=34, "On Boot - Limit Disabled - Reverse"=35, "Fault - Over Temp"=41, "Fault - Under Voltage"=42, "Fault - Forward Limit"=43, "Fault - Reverse Limit"=44, "Fault - Hardware Failure"=45, "Fault - Forward Soft Limit"=46, "Fault - Reverse Soft Limit"=47, "Sticky Fault - Over Temp"=48, "Sticky Fault - Under Voltage"=49, "Sticky Fault - Forward Limit"=50, "Sticky Fault - Reverse Limit"=51, "Sticky Fault - Forward Soft Limit"=52, "Sticky Fault - Reverse Soft Limit"=53, "Applied Throttle"=61, "Closed-Loop Error"=62, "Select Feedback Device"=63, "Reverse Closed-Loop Output"=64, "Mode Select"=65, "Profile Slot Select"=66, "Ramp Throttle"=67, "Reverse Feedback Sensor"=68, "Limit Switch Enabled"=69, "Limit Switch Closed - Forward"=70, "Limit Switch Closed - Reverse"=71, "Sensor Position"=73, "Sensor Velocity"=74, "Current"=75, "Brake is Enabled"=76, "Encoder Position"=77, "Encoder Velocity"=78, "Encoder Index Rise Events"=79, "Encoder A Pin State"=80, "Encoder B Pin State"=81, "Encoder Index Pin State"=82, "Analog In with Overflow"=83, "Analog In Velocity"=84, "Temperature"=85, "Battery Voltage"=86, "Reset Count"=87, "Reset Flags"=88, "Firmware Version"=89, "Settings Changed"=90, "Quad Filter Enable"=91, "Ignore Disable Broadcast"=92, "I Accumulator"=93, "Status 1 Frame Rate Ms"=94, "Status 2 Frame Rate Ms"=95, "Status 3 Frame Rate Ms"=96, "Status 4 Frame Rate Ms"=97, "Status 6 Frame Rate Ms"=98, "Status 7 Frame Rate Ms"=99, "Enable Index Pin Clear Position"=100, "Peak Positive Output"=104, "Nominal Positive Output"=105, "Peak Negative Output"=106, "Nominal Negative Output"=107, "Quad Index Pin Polarity"=108, "Status 8 Frame Rate Ms"=109, "Allow Position Overflow"=110, "Slot 0 - Allowable Closed-Loop Error"=111, "Number Potentiometer Turns"=112, "Encoder Codes Per Rev"=113, "Pulse Width Decoded Position"=114, "Analog Position"=115, "Voltage Compensation Rate (V/s)"=116, "Slot 1 - Allowable Closed-Loop Error"=117, "Motion Profile Has Underrun Err"=119, "Reserved 120"=120, "Legacy Control Mode"=121, "Motion Magic Acceleration"=122, "Motion Magic Cruise Velocity"=123, "Status 10 Frame Rate"=124, "Current Limit Threshold"=125, "CustomParam0"=137, "CustomParam1"=138, "PersStorageSaving"=139, "ClearPositionOnLimitF"=144, "ClearPositionOnLimitR"=145, "NominalBatteryVoltage"=146, "SampleVelocityPeriod"=147, "SampleVelocityWindow"=148] ("Parameter")
          n48 = Unbundle By Name(w95) -> ("CAN.Device Number"=w98:u8)
          n49 = call <vilib>:"WPI_CANTalonSRX_SetParameter.vi"("Value"=0.0, "Parameter"=w97, "Device ID (0)"=w98) -> ()  [unwired: 7 in, 2 out]
        }
        frame #5 {
          n50 = while {
            tunnel: w100 -> [w102]
            tunnel: [w101] -> w99
            stop <- w105 stop-if-true
            n51 = call <vilib>:"WPI_CANTalonSRX_GetStatus.vi"("CAN Talon SRX Ref"=w102) -> ("Talon SRX Status"=w108:T15, "CAN Talon SRX Ref"=w107:T7)  [unwired: 8 in, 1 out]
            n52 = Unbundle By Name(w108) -> ("Encoder Position"=w104:dbl)
            "Encoder Position 3" <- w104
            n53 = Less?(x=500000.0, y=w104) -> (x < y?=w105:bool)
            n54 = case shown="False" w105 {
              tunnel: [-0.5 ("x") 0.0 ("x")] -> w106
              frame False {
              }
              frame True {
              }
            }
            n55 = call <vilib>:"WPI_MotorControlSetOutput.vi"("Output"=w106, "MotorControlDevRef"=w107) -> ("MotorControlDevRef"=w101:T7)  [unwired: 7 in, 2 out]
          }
        }
        frame #6 {
          w113 = T14 77 items=["Slot 0 - P"=1, "Slot 0 - I"=2, "Slot 0 - D"=3, "Slot 0 - F"=4, "Slot 0 - I Zone"=5, "Slot 0 - Ramp Rate"=6, "Slot 1 - P"=11, "Slot 1 - I"=12, "Slot 1 - D"=13, "Slot 1 - F"=14, "Slot 1 - I Zone"=15, "Slot 1 - Ramp Rate"=16, "Soft Limit - Forward"=21, "Soft Limit - Reverse"=22, "Soft Limit - Forward Enable"=23, "Soft Limit - Reverse Enable"=24, "On Boot - Brake Mode"=31, "On Boot - Limit Normally Closed - Forward"=32, "On Boot - Limit Normally Closed - Reverse"=33, "On Boot - Limit Disabled - Forward"=34, "On Boot - Limit Disabled - Reverse"=35, "Fault - Over Temp"=41, "Fault - Under Voltage"=42, "Fault - Forward Limit"=43, "Fault - Reverse Limit"=44, "Fault - Hardware Failure"=45, "Fault - Forward Soft Limit"=46, "Fault - Reverse Soft Limit"=47, "Sticky Fault - Over Temp"=48, "Sticky Fault - Under Voltage"=49, "Sticky Fault - Forward Limit"=50, "Sticky Fault - Reverse Limit"=51, "Sticky Fault - Forward Soft Limit"=52, "Sticky Fault - Reverse Soft Limit"=53, "Applied Throttle"=61, "Closed-Loop Error"=62, "Select Feedback Device"=63, "Reverse Closed-Loop Output"=64, "Mode Select"=65, "Profile Slot Select"=66, "Ramp Throttle"=67, "Reverse Feedback Sensor"=68, "Limit Switch Enabled"=69, "Limit Switch Closed - Forward"=70, "Limit Switch Closed - Reverse"=71, "Sensor Position"=73, "Sensor Velocity"=74, "Current"=75, "Brake is Enabled"=76, "Encoder Position"=77, "Encoder Velocity"=78, "Encoder Index Rise Events"=79, "Encoder A Pin State"=80, "Encoder B Pin State"=81, "Encoder Index Pin State"=82, "Analog In with Overflow"=83, "Analog In Velocity"=84, "Temperature"=85, "Battery Voltage"=86, "Reset Count"=87, "Reset Flags"=88, "Firmware Version"=89, "Settings Changed"=90, "Quad Filter Enable"=91, "Ignore Disable Broadcast"=92, "I Accumulator"=93, "Status 1 Frame Rate Ms"=94, "Status 2 Frame Rate Ms"=95, "Status 3 Frame Rate Ms"=96, "Status 4 Frame Rate Ms"=97, "Status 6 Frame Rate Ms"=98, "Status 7 Frame Rate Ms"=99, "Enable Index Pin Clear Position"=100, "Peak Positive Output"=104, "Nominal Positive Output"=105, "Peak Negative Output"=106, "Nominal Negative Output"=107, "Quad Index Pin Polarity"=108, "Status 8 Frame Rate Ms"=109, "Allow Position Overflow"=110, "Slot 0 - Allowable Closed-Loop Error"=111, "Number Potentiometer Turns"=112, "Encoder Codes Per Rev"=113, "Pulse Width Decoded Position"=114, "Analog Position"=115, "Voltage Compensation Rate (V/s)"=116, "Slot 1 - Allowable Closed-Loop Error"=117, "Motion Profile Has Underrun Err"=119, "Reserved 120"=120, "Legacy Control Mode"=121, "Motion Magic Acceleration"=122, "Motion Magic Cruise Velocity"=123, "Status 10 Frame Rate"=124, "Current Limit Threshold"=125, "CustomParam0"=137, "CustomParam1"=138, "PersStorageSaving"=139, "ClearPositionOnLimitF"=144, "ClearPositionOnLimitR"=145, "NominalBatteryVoltage"=146, "SampleVelocityPeriod"=147, "SampleVelocityWindow"=148] ("Parameter")
          n56 = Unbundle By Name(w111) -> ("CAN.Device Number"=w112:u8)
          n57 = call <vilib>:"WPI_CANTalonSRX_SetParameter.vi"("Value"=0.0, "Parameter"=w113, "Device ID (0)"=w112) -> ()  [unwired: 7 in, 2 out]
        }
        frame #7 {
          n58 = while {
            tunnel: w116 -> [w118]
            tunnel: [w117] -> w115
            stop <- w121 stop-if-true
            n59 = call <vilib>:"WPI_CANTalonSRX_GetStatus.vi"("CAN Talon SRX Ref"=w118) -> ("Talon SRX Status"=w124:T15, "CAN Talon SRX Ref"=w123:T7)  [unwired: 8 in, 1 out]
            n60 = Unbundle By Name(w124) -> ("Encoder Position"=w120:dbl)
            "Encoder Position 4" <- w120
            n61 = Greater?(x=-20000.0, y=w120) -> (0:w121:bool)
            n62 = case shown="False" w121 {
              tunnel: [0.3 ("x") 0.0 ("x")] -> w122
              frame False {
              }
              frame True {
              }
            }
            n63 = call <vilib>:"WPI_MotorControlSetOutput.vi"("Output"=w122, "MotorControlDevRef"=w123) -> ("MotorControlDevRef"=w117:T7)  [unwired: 7 in, 2 out]
          }
        }
        frame #8 {
          w129 = T14 77 items=["Slot 0 - P"=1, "Slot 0 - I"=2, "Slot 0 - D"=3, "Slot 0 - F"=4, "Slot 0 - I Zone"=5, "Slot 0 - Ramp Rate"=6, "Slot 1 - P"=11, "Slot 1 - I"=12, "Slot 1 - D"=13, "Slot 1 - F"=14, "Slot 1 - I Zone"=15, "Slot 1 - Ramp Rate"=16, "Soft Limit - Forward"=21, "Soft Limit - Reverse"=22, "Soft Limit - Forward Enable"=23, "Soft Limit - Reverse Enable"=24, "On Boot - Brake Mode"=31, "On Boot - Limit Normally Closed - Forward"=32, "On Boot - Limit Normally Closed - Reverse"=33, "On Boot - Limit Disabled - Forward"=34, "On Boot - Limit Disabled - Reverse"=35, "Fault - Over Temp"=41, "Fault - Under Voltage"=42, "Fault - Forward Limit"=43, "Fault - Reverse Limit"=44, "Fault - Hardware Failure"=45, "Fault - Forward Soft Limit"=46, "Fault - Reverse Soft Limit"=47, "Sticky Fault - Over Temp"=48, "Sticky Fault - Under Voltage"=49, "Sticky Fault - Forward Limit"=50, "Sticky Fault - Reverse Limit"=51, "Sticky Fault - Forward Soft Limit"=52, "Sticky Fault - Reverse Soft Limit"=53, "Applied Throttle"=61, "Closed-Loop Error"=62, "Select Feedback Device"=63, "Reverse Closed-Loop Output"=64, "Mode Select"=65, "Profile Slot Select"=66, "Ramp Throttle"=67, "Reverse Feedback Sensor"=68, "Limit Switch Enabled"=69, "Limit Switch Closed - Forward"=70, "Limit Switch Closed - Reverse"=71, "Sensor Position"=73, "Sensor Velocity"=74, "Current"=75, "Brake is Enabled"=76, "Encoder Position"=77, "Encoder Velocity"=78, "Encoder Index Rise Events"=79, "Encoder A Pin State"=80, "Encoder B Pin State"=81, "Encoder Index Pin State"=82, "Analog In with Overflow"=83, "Analog In Velocity"=84, "Temperature"=85, "Battery Voltage"=86, "Reset Count"=87, "Reset Flags"=88, "Firmware Version"=89, "Settings Changed"=90, "Quad Filter Enable"=91, "Ignore Disable Broadcast"=92, "I Accumulator"=93, "Status 1 Frame Rate Ms"=94, "Status 2 Frame Rate Ms"=95, "Status 3 Frame Rate Ms"=96, "Status 4 Frame Rate Ms"=97, "Status 6 Frame Rate Ms"=98, "Status 7 Frame Rate Ms"=99, "Enable Index Pin Clear Position"=100, "Peak Positive Output"=104, "Nominal Positive Output"=105, "Peak Negative Output"=106, "Nominal Negative Output"=107, "Quad Index Pin Polarity"=108, "Status 8 Frame Rate Ms"=109, "Allow Position Overflow"=110, "Slot 0 - Allowable Closed-Loop Error"=111, "Number Potentiometer Turns"=112, "Encoder Codes Per Rev"=113, "Pulse Width Decoded Position"=114, "Analog Position"=115, "Voltage Compensation Rate (V/s)"=116, "Slot 1 - Allowable Closed-Loop Error"=117, "Motion Profile Has Underrun Err"=119, "Reserved 120"=120, "Legacy Control Mode"=121, "Motion Magic Acceleration"=122, "Motion Magic Cruise Velocity"=123, "Status 10 Frame Rate"=124, "Current Limit Threshold"=125, "CustomParam0"=137, "CustomParam1"=138, "PersStorageSaving"=139, "ClearPositionOnLimitF"=144, "ClearPositionOnLimitR"=145, "NominalBatteryVoltage"=146, "SampleVelocityPeriod"=147, "SampleVelocityWindow"=148] ("Parameter")
          n64 = Unbundle By Name(w127) -> ("CAN.Device Number"=w128:u8)
          n65 = call <vilib>:"WPI_CANTalonSRX_SetParameter.vi"("Value"=0.0, "Parameter"=w129, "Device ID (0)"=w128) -> ()  [unwired: 7 in, 2 out]
        }
      }
    }
    frame "SHOOT" {
      n66 = call-poly <vilib>:"WPI_RobotDriveArcadeDrive.vi"("error in (no error)"=w155, "Y axis value"=0.0, "X axis value"=0.0, "RobotDriveDevRef"=w156) -> ("error out"=w152:errorcluster, "RobotDriveDevRef"=w153:T11)  [unwired: 5 in, 1 out]
      n67 = call <vilib>:"WPI_RobotDriveDelayAndUpdateSafety.vi"("error in (no error)"=w152, "Delay (s)"=2.0, "RobotDriveDevRef"=w153) -> ("error out"=w148:errorcluster, "RobotDriveDevRef 2"=w149:T11)  [unwired: 7 in]
      n68 = call-poly <vilib>:"WPI_RobotDriveArcadeDrive.vi"("error in (no error)"=w148, "Y axis value"=0.85, "RobotDriveDevRef"=w149) -> ("error out"=w145:errorcluster, "RobotDriveDevRef"=w146:T11)  [unwired: 6 in, 1 out]
      n69 = call <vilib>:"WPI_RobotDriveDelayAndUpdateSafety.vi"("error in (no error)"=w145, "Delay (s)"=1.25, "RobotDriveDevRef"=w146) -> ("error out"=w134:errorcluster, "RobotDriveDevRef 2"=w135:T11)  [unwired: 7 in]
      n70 = call-poly <vilib>:"WPI_RobotDriveArcadeDrive.vi"("error in (no error)"=w134, "Y axis value"=0.0, "RobotDriveDevRef"=w135) -> ("error out"=w137:errorcluster, "RobotDriveDevRef"=w136:T11)  [unwired: 6 in, 1 out]
      n71 = call <vilib>:"WPI_RobotDriveDelayAndUpdateSafety.vi"("error in (no error)"=w137, "Delay (s)"=0.1, "RobotDriveDevRef"=w136) -> ("error out"=w132:errorcluster, "RobotDriveDevRef 2"=w131:T11)  [unwired: 7 in]
      n72 = Merge Errors(w143, w142) -> (w141:errorcluster)
      n73 = Merge Errors(w132, w141) -> (w140:errorcluster)
      n74 = call <vilib>:"WPI_CANTalonSRX_SetReference.vi"("error in (no error)"=w140, "Feedback Reference"=WPI_CANTalonSRX_APIFeedbackSelect."CTR Magnetic Enc (Relative)", "CAN Talon SRX Ref"=w186) -> ("error out"=w185:errorcluster, "CAN Talon SRX Ref"=w194:T7)  [unwired: 7 in]
      n75 = call <vilib>:"WPI_MotorControlSetOutput.vi"("error in (no error)"=w140, "Output"=0.75, "MotorControlDevRef"=w173) -> ("error out"=w170:errorcluster, "MotorControlDevRef"=w168:T7)  [unwired: 6 in, 1 out]
      n76 = call <vilib>:"WPI_CANTalonSRX_SetPID.vi"("CAN Talon SRX Ref"=w194, "P"=0.0, "I"=0.0, "D"=0.0, "error in (no error)"=w185, "F"=0.01, "I Zone"=0.0, "Ramp Rate"=0.0) -> ("CAN Talon SRX Ref"=w191:T7, "error out"=w184:errorcluster)  [unwired: 6 in]
      n77 = call <vilib>:"WPI_CANTalonSRX_ChangeMode.vi"("error in (no error)"=w184, "Output"=9800.0 ("y"), "Control Mode"=WPI_CANTalonSRX_APIControlMode."Speed", "CAN Talon SRX Ref"=w191) -> ("error out"=w183:errorcluster, "CAN Talon SRX Ref"=w187:T7)  [unwired: 6 in]
      n78 = call <vilib>:"WPI_CANTalonSRX_GetStatus.vi"("error in (no error)"=w183, "CAN Talon SRX Ref"=w187) -> ("error out"=w171:errorcluster)  [unwired: 7 in, 2 out]
      n79 = Merge Errors(w171, w170) -> (w169:errorcluster)
      n80 = call <vilib>:"WPI_RobotDriveDelayAndUpdateSafety.vi"("error in (no error)"=w169, "Delay (s)"=9.0, "RobotDriveDevRef"=w131) -> ("error out"=w167:errorcluster, "RobotDriveDevRef 2"=w182:T11)  [unwired: 7 in]
      n81 = call <vilib>:"WPI_MotorControlSetOutput.vi"("error in (no error)"=w167, "Output"=0.0, "MotorControlDevRef"=w168) -> ("error out"=w139:errorcluster)  [unwired: 6 in, 2 out]
      n82 = call-poly <vilib>:"WPI_RobotDriveArcadeDrive.vi"("error in (no error)"=w139, "Y axis value"=0.0, "X axis value"=0.4, "RobotDriveDevRef"=w182) -> ("error out"=w179:errorcluster, "RobotDriveDevRef"=w180:T11)  [unwired: 5 in, 1 out]
      n83 = call <vilib>:"WPI_RobotDriveDelayAndUpdateSafety.vi"("error in (no error)"=w179, "Delay (s)"=1.0, "RobotDriveDevRef"=w180) -> ("error out"=w160:errorcluster, "RobotDriveDevRef 2"=w159:T11)  [unwired: 7 in]
      n84 = call-poly <vilib>:"WPI_RobotDriveArcadeDrive.vi"("error in (no error)"=w160, "Y axis value"=-0.8, "X axis value"=0.0, "RobotDriveDevRef"=w159) -> ("error out"=w163:errorcluster, "RobotDriveDevRef"=w164:T11)  [unwired: 5 in, 1 out]
      n85 = call <vilib>:"WPI_RobotDriveDelayAndUpdateSafety.vi"("error in (no error)"=w163, "Delay (s)"=2.25, "RobotDriveDevRef"=w164) -> ("error out"=w157:errorcluster, "RobotDriveDevRef 2"=w158:T11)  [unwired: 7 in]
      n86 = call-poly <vilib>:"WPI_RobotDriveArcadeDrive.vi"("error in (no error)"=w157, "Y axis value"=0.0, "X axis value"=0.0, "RobotDriveDevRef"=w158) -> ()  [unwired: 5 in, 3 out]
    }
    frame "SHOOT2" {
      n87 = call-poly <vilib>:"WPI_RobotDriveArcadeDrive.vi"("error in (no error)"=w232, "Y axis value"=0.0, "X axis value"=0.0, "RobotDriveDevRef"=w231) -> ("error out"=w230:errorcluster, "RobotDriveDevRef"=w229:T11)  [unwired: 5 in, 1 out]
      n88 = call <vilib>:"WPI_RobotDriveDelayAndUpdateSafety.vi"("error in (no error)"=w230, "Delay (s)"=2.0, "RobotDriveDevRef"=w229) -> ("error out"=w225:errorcluster, "RobotDriveDevRef 2"=w224:T11)  [unwired: 7 in]
      n89 = call-poly <vilib>:"WPI_RobotDriveArcadeDrive.vi"("error in (no error)"=w225, "Y axis value"=0.57, "RobotDriveDevRef"=w224) -> ("error out"=w221:errorcluster, "RobotDriveDevRef"=w222:T11)  [unwired: 6 in, 1 out]
      n90 = call <vilib>:"WPI_RobotDriveDelayAndUpdateSafety.vi"("error in (no error)"=w221, "Delay (s)"=1.0, "RobotDriveDevRef"=w222) -> ("error out"=w219:errorcluster, "RobotDriveDevRef 2"=w218:T11)  [unwired: 7 in]
      n91 = call-poly <vilib>:"WPI_RobotDriveArcadeDrive.vi"("error in (no error)"=w219, "X axis value"=-0.5, "RobotDriveDevRef"=w218) -> ("error out"=w216:errorcluster, "RobotDriveDevRef"=w217:T11)  [unwired: 6 in, 1 out]
      n92 = Merge Errors(w212, w211) -> (w210:errorcluster)
      n93 = call <vilib>:"WPI_RobotDriveDelayAndUpdateSafety.vi"("error in (no error)"=w216, "Delay (s)"=0.25, "RobotDriveDevRef"=w217) -> ("error out"=w204:errorcluster, "RobotDriveDevRef 2"=w205:T11)  [unwired: 7 in]
      n94 = call-poly <vilib>:"WPI_RobotDriveArcadeDrive.vi"("error in (no error)"=w204, "Y axis value"=0.0, "X axis value"=0.0, "RobotDriveDevRef"=w205) -> ("error out"=w207:errorcluster, "RobotDriveDevRef"=w206:T11)  [unwired: 5 in, 1 out]
      n95 = call <vilib>:"WPI_RobotDriveDelayAndUpdateSafety.vi"("error in (no error)"=w207, "Delay (s)"=0.1, "RobotDriveDevRef"=w206) -> ("error out"=w199:errorcluster, "RobotDriveDevRef 2"=w200:T11)  [unwired: 7 in]
      n96 = Merge Errors(w199, w210) -> (w209:errorcluster)
      n97 = call <vilib>:"WPI_CANTalonSRX_SetReference.vi"("error in (no error)"=w209, "Feedback Reference"=WPI_CANTalonSRX_APIFeedbackSelect."CTR Magnetic Enc (Relative)", "CAN Talon SRX Ref"=w214) -> ("error out"=w281:errorcluster, "CAN Talon SRX Ref"=w289:T7)  [unwired: 7 in]
      n98 = call <vilib>:"WPI_MotorControlSetOutput.vi"("error in (no error)"=w209, "Output"=0.75, "MotorControlDevRef"=w213) -> ("error out"=w269:errorcluster, "MotorControlDevRef"=w267:T7)  [unwired: 6 in, 1 out]
      n99 = call <vilib>:"WPI_CANTalonSRX_SetPID.vi"("CAN Talon SRX Ref"=w289, "P"=0.0, "I"=0.0, "D"=0.0, "error in (no error)"=w281, "F"=0.01, "I Zone"=0.0, "Ramp Rate"=0.0) -> ("CAN Talon SRX Ref"=w286:T7, "error out"=w280:errorcluster)  [unwired: 6 in]
      n100 = call <vilib>:"WPI_CANTalonSRX_ChangeMode.vi"("error in (no error)"=w280, "Output"=9800.0 ("y"), "Control Mode"=WPI_CANTalonSRX_APIControlMode."Speed", "CAN Talon SRX Ref"=w286) -> ("error out"=w279:errorcluster, "CAN Talon SRX Ref"=w282:T7)  [unwired: 6 in]
      n101 = call <vilib>:"WPI_CANTalonSRX_GetStatus.vi"("error in (no error)"=w279, "CAN Talon SRX Ref"=w282) -> ("error out"=w270:errorcluster, "CAN Talon SRX Ref"=w252:T7)  [unwired: 7 in, 1 out]
      n102 = Merge Errors(w270, w269) -> (w268:errorcluster)
      n103 = call <vilib>:"WPI_RobotDriveDelayAndUpdateSafety.vi"("error in (no error)"=w268, "Delay (s)"=9.0, "RobotDriveDevRef"=w200) -> ("error out"=w251:errorcluster, "RobotDriveDevRef 2"=w278:T11)  [unwired: 7 in]
      n104 = call <vilib>:"WPI_CANTalonSRX_ChangeMode.vi"("error in (no error)"=w251, "Output"=0.0 ("y"), "Control Mode"=WPI_CANTalonSRX_APIControlMode."Speed", "CAN Talon SRX Ref"=w252) -> ("error out"=w253:errorcluster, "CAN Talon SRX Ref"=w254:T7)  [unwired: 6 in]
      n105 = call <vilib>:"WPI_MotorControlSetOutput.vi"("error in (no error)"=w251, "Output"=0.0, "MotorControlDevRef"=w267) -> ("error out"=w249:errorcluster)  [unwired: 6 in, 2 out]
      n106 = call <vilib>:"WPI_CANTalonSRX_GetStatus.vi"("error in (no error)"=w253, "CAN Talon SRX Ref"=w254) -> ("error out"=w250:errorcluster)  [unwired: 7 in, 2 out]
      n107 = Merge Errors(w250, w249) -> (w248:errorcluster)
      n108 = call <vilib>:"WPI_RobotDriveTankDrive.vi"("error in (no error)"=w248, "Right axis value"=0.6 ("Y axis value"), "Left axis value"=0.6, "RobotDriveDevRef"=w278) -> ("error out"=w276:errorcluster, "RobotDriveDevRef"=w277:T11)  [unwired: 5 in, 1 out]
      n109 = call <vilib>:"WPI_RobotDriveDelayAndUpdateSafety.vi"("error in (no error)"=w276, "Delay (s)"=0.25, "RobotDriveDevRef"=w277) -> ("error out"=w260:errorcluster, "RobotDriveDevRef 2"=w259:T11)  [unwired: 7 in]
      n110 = call-poly <vilib>:"WPI_RobotDriveArcadeDrive.vi"("error in (no error)"=w260, "Y axis value"=0.0, "X axis value"=-0.8, "RobotDriveDevRef"=w259) -> ("error out"=w263:errorcluster, "RobotDriveDevRef"=w264:T11)  [unwired: 5 in, 1 out]
      n111 = call <vilib>:"WPI_RobotDriveDelayAndUpdateSafety.vi"("error in (no error)"=w263, "Delay (s)"=0.5, "RobotDriveDevRef"=w264) -> ("error out"=w257:errorcluster, "RobotDriveDevRef 2"=w258:T11)  [unwired: 7 in]
      n112 = call-poly <vilib>:"WPI_RobotDriveArcadeDrive.vi"("error in (no error)"=w257, "Y axis value"=-0.65, "X axis value"=-0.5, "RobotDriveDevRef"=w258) -> ("error out"=w246:errorcluster, "RobotDriveDevRef"=w247:T11)  [unwired: 5 in, 1 out]
      n113 = call <vilib>:"WPI_RobotDriveDelayAndUpdateSafety.vi"("error in (no error)"=w246, "Delay (s)"=1.0, "RobotDriveDevRef"=w247) -> ("error out"=w244:errorcluster, "RobotDriveDevRef 2"=w243:T11)  [unwired: 7 in]
      n114 = call-poly <vilib>:"WPI_RobotDriveArcadeDrive.vi"("error in (no error)"=w244, "Y axis value"=-0.5 ("X axis value"), "RobotDriveDevRef"=w243) -> ("error out"=w238:errorcluster, "RobotDriveDevRef"=w239:T11)  [unwired: 6 in, 1 out]
      n115 = call <vilib>:"WPI_RobotDriveDelayAndUpdateSafety.vi"("error in (no error)"=w238, "Delay (s)"=2.0, "RobotDriveDevRef"=w239) -> ("error out"=w235:errorcluster, "RobotDriveDevRef 2"=w236:T11)  [unwired: 7 in]
      n116 = call-poly <vilib>:"WPI_RobotDriveArcadeDrive.vi"("error in (no error)"=w235, "Y axis value"=0.0, "X axis value"=0.0, "RobotDriveDevRef"=w236) -> ()  [unwired: 5 in, 3 out]
    }
    frame "SHOOTBLUE" {
      n117 = call <vilib>:"WPI_CANTalonSRX_SetReference.vi"("error in (no error)"=w295, "Feedback Reference"=WPI_CANTalonSRX_APIFeedbackSelect."CTR Magnetic Enc (Relative)", "CAN Talon SRX Ref"=w294) -> ("error out"=w327:errorcluster, "CAN Talon SRX Ref"=w335:T7)  [unwired: 7 in]
      n118 = call <vilib>:"WPI_MotorControlSetOutput.vi"("error in (no error)"=w296, "Output"=0.75, "MotorControlDevRef"=w297) -> ("error out"=w313:errorcluster, "MotorControlDevRef"=w311:T7)  [unwired: 6 in, 1 out]
      n119 = call <vilib>:"WPI_CANTalonSRX_SetPID.vi"("CAN Talon SRX Ref"=w335, "P"=0.0, "I"=0.0, "D"=0.0, "error in (no error)"=w327, "F"=0.01, "I Zone"=0.0, "Ramp Rate"=0.0) -> ("CAN Talon SRX Ref"=w332:T7, "error out"=w326:errorcluster)  [unwired: 6 in]
      n120 = call <vilib>:"WPI_CANTalonSRX_ChangeMode.vi"("error in (no error)"=w326, "Output"=9800.0 ("y"), "Control Mode"=WPI_CANTalonSRX_APIControlMode."Speed", "CAN Talon SRX Ref"=w332) -> ("error out"=w325:errorcluster, "CAN Talon SRX Ref"=w328:T7)  [unwired: 6 in]
      n121 = call <vilib>:"WPI_CANTalonSRX_GetStatus.vi"("error in (no error)"=w325, "CAN Talon SRX Ref"=w328) -> ("error out"=w314:errorcluster)  [unwired: 7 in, 2 out]
      n122 = Merge Errors(w314, w313) -> (w312:errorcluster)
      n123 = call <vilib>:"WPI_RobotDriveDelayAndUpdateSafety.vi"("error in (no error)"=w312, "Delay (s)"=10.0, "RobotDriveDevRef"=w298) -> ("error out"=w310:errorcluster, "RobotDriveDevRef 2"=w324:T11)  [unwired: 7 in]
      n124 = call <vilib>:"WPI_MotorControlSetOutput.vi"("error in (no error)"=w310, "Output"=0.0, "MotorControlDevRef"=w311) -> ("error out"=w299:errorcluster)  [unwired: 6 in, 2 out]
      n125 = call-poly <vilib>:"WPI_RobotDriveArcadeDrive.vi"("error in (no error)"=w299, "Y axis value"=0.0, "X axis value"=0.4, "RobotDriveDevRef"=w324) -> ("error out"=w321:errorcluster, "RobotDriveDevRef"=w322:T11)  [unwired: 5 in, 1 out]
      n126 = call <vilib>:"WPI_RobotDriveDelayAndUpdateSafety.vi"("error in (no error)"=w321, "Delay (s)"=1.0, "RobotDriveDevRef"=w322) -> ("error out"=w303:errorcluster, "RobotDriveDevRef 2"=w302:T11)  [unwired: 7 in]
      n127 = call-poly <vilib>:"WPI_RobotDriveArcadeDrive.vi"("error in (no error)"=w303, "Y axis value"=-0.6, "X axis value"=0.25, "RobotDriveDevRef"=w302) -> ("error out"=w306:errorcluster, "RobotDriveDevRef"=w307:T11)  [unwired: 5 in, 1 out]
      n128 = call <vilib>:"WPI_RobotDriveDelayAndUpdateSafety.vi"("error in (no error)"=w306, "Delay (s)"=3.0, "RobotDriveDevRef"=w307) -> ("error out"=w300:errorcluster, "RobotDriveDevRef 2"=w301:T11)  [unwired: 7 in]
      n129 = call-poly <vilib>:"WPI_RobotDriveArcadeDrive.vi"("error in (no error)"=w300, "Y axis value"=0.0, "X axis value"=0.0, "RobotDriveDevRef"=w301) -> ()  [unwired: 5 in, 3 out]
    }
    frame "SHOOTRED" {
      # "SHOOTRED"
      n130 = call <vilib>:"WPI_CANTalonSRX_SetReference.vi"("error in (no error)"=w392, "Feedback Reference"=WPI_CANTalonSRX_APIFeedbackSelect."CTR Magnetic Enc (Relative)", "CAN Talon SRX Ref"=w393) -> ("error out"=w391:errorcluster, "CAN Talon SRX Ref"=w401:T7)  [unwired: 7 in]
      n131 = call <vilib>:"WPI_MotorControlSetOutput.vi"("error in (no error)"=w379, "Output"=0.75, "MotorControlDevRef"=w380) -> ("error out"=w376:errorcluster, "MotorControlDevRef"=w374:T7)  [unwired: 6 in, 1 out]
      n132 = call <vilib>:"WPI_CANTalonSRX_SetPID.vi"("CAN Talon SRX Ref"=w401, "P"=0.0, "I"=0.0, "D"=0.0, "error in (no error)"=w391, "F"=0.01, "I Zone"=0.0, "Ramp Rate"=0.0) -> ("CAN Talon SRX Ref"=w398:T7, "error out"=w390:errorcluster)  [unwired: 6 in]
      n133 = call <vilib>:"WPI_CANTalonSRX_ChangeMode.vi"("error in (no error)"=w390, "Output"=9800.0 ("y"), "Control Mode"=WPI_CANTalonSRX_APIControlMode."Speed", "CAN Talon SRX Ref"=w398) -> ("error out"=w389:errorcluster, "CAN Talon SRX Ref"=w394:T7)  [unwired: 6 in]
      n134 = call <vilib>:"WPI_CANTalonSRX_GetStatus.vi"("error in (no error)"=w389, "CAN Talon SRX Ref"=w394) -> ("error out"=w377:errorcluster, "CAN Talon SRX Ref"=w359:T7)  [unwired: 7 in, 1 out]
      n135 = Merge Errors(w377, w376) -> (w375:errorcluster)
      n136 = call <vilib>:"WPI_RobotDriveDelayAndUpdateSafety.vi"("error in (no error)"=w375, "Delay (s)"=10.0, "RobotDriveDevRef"=w387) -> ("error out"=w358:errorcluster, "RobotDriveDevRef 2"=w388:T11)  [unwired: 7 in]
      n137 = call <vilib>:"WPI_CANTalonSRX_ChangeMode.vi"("error in (no error)"=w358, "Output"=0.0 ("y"), "Control Mode"=WPI_CANTalonSRX_APIControlMode."Speed", "CAN Talon SRX Ref"=w359) -> ("error out"=w360:errorcluster, "CAN Talon SRX Ref"=w361:T7)  [unwired: 6 in]
      n138 = call <vilib>:"WPI_MotorControlSetOutput.vi"("error in (no error)"=w358, "Output"=0.0, "MotorControlDevRef"=w374) -> ("error out"=w356:errorcluster)  [unwired: 6 in, 2 out]
      n139 = call <vilib>:"WPI_CANTalonSRX_GetStatus.vi"("error in (no error)"=w360, "CAN Talon SRX Ref"=w361) -> ("error out"=w357:errorcluster)  [unwired: 7 in, 2 out]
      n140 = Merge Errors(w357, w356) -> (w355:errorcluster)
      n141 = call <vilib>:"WPI_RobotDriveTankDrive.vi"("error in (no error)"=w355, "Right axis value"=0.6 ("Y axis value"), "Left axis value"=0.6, "RobotDriveDevRef"=w388) -> ("error out"=w385:errorcluster, "RobotDriveDevRef"=w386:T11)  [unwired: 5 in, 1 out]
      n142 = call <vilib>:"WPI_RobotDriveDelayAndUpdateSafety.vi"("error in (no error)"=w385, "Delay (s)"=0.25, "RobotDriveDevRef"=w386) -> ("error out"=w367:errorcluster, "RobotDriveDevRef 2"=w366:T11)  [unwired: 7 in]
      n143 = call-poly <vilib>:"WPI_RobotDriveArcadeDrive.vi"("error in (no error)"=w367, "Y axis value"=0.0, "X axis value"=-0.8, "RobotDriveDevRef"=w366) -> ("error out"=w370:errorcluster, "RobotDriveDevRef"=w371:T11)  [unwired: 5 in, 1 out]
      n144 = call <vilib>:"WPI_RobotDriveDelayAndUpdateSafety.vi"("error in (no error)"=w370, "Delay (s)"=0.5, "RobotDriveDevRef"=w371) -> ("error out"=w364:errorcluster, "RobotDriveDevRef 2"=w365:T11)  [unwired: 7 in]
      n145 = call-poly <vilib>:"WPI_RobotDriveArcadeDrive.vi"("error in (no error)"=w364, "Y axis value"=-0.5, "X axis value"=-0.55, "RobotDriveDevRef"=w365) -> ("error out"=w353:errorcluster, "RobotDriveDevRef"=w354:T11)  [unwired: 5 in, 1 out]
      n146 = call <vilib>:"WPI_RobotDriveDelayAndUpdateSafety.vi"("error in (no error)"=w353, "Delay (s)"=1.0, "RobotDriveDevRef"=w354) -> ("error out"=w351:errorcluster, "RobotDriveDevRef 2"=w350:T11)  [unwired: 7 in]
      n147 = call-poly <vilib>:"WPI_RobotDriveArcadeDrive.vi"("error in (no error)"=w351, "Y axis value"=-0.5 ("X axis value"), "RobotDriveDevRef"=w350) -> ("error out"=w345:errorcluster, "RobotDriveDevRef"=w346:T11)  [unwired: 6 in, 1 out]
      n148 = call <vilib>:"WPI_RobotDriveDelayAndUpdateSafety.vi"("error in (no error)"=w345, "Delay (s)"=2.0, "RobotDriveDevRef"=w346) -> ("error out"=w342:errorcluster, "RobotDriveDevRef 2"=w343:T11)  [unwired: 7 in]
      n149 = call-poly <vilib>:"WPI_RobotDriveArcadeDrive.vi"("error in (no error)"=w342, "Y axis value"=0.0, "X axis value"=0.0, "RobotDriveDevRef"=w343) -> ()  [unwired: 5 in, 3 out]
    }
    frame "NEW" {
      n150 = while {
        tunnel: w427 -> [w519]
        tunnel: w426 -> [w518]
        tunnel: [w512] -> w428
        tunnel: [w511] -> w429
        tunnel: w425 -> [w510]
        tunnel: w424 -> [w504]
        tunnel: [w500] -> w423
        tunnel: [w499] -> w422
        tunnel: w413 -> [w498]
        tunnel: [w498] -> w412
        stop <- w501 stop-if-true
        n151 = call <vilib>:"WPI_EncoderGet.vi"("EncoderDevRef"=w510) -> ("Distance"=w509:dbl, "EncoderDevRef"=w500:T3)  [unwired: 5 in, 4 out]
        n152 = call <vilib>:"WPI_EncoderGet.vi"("EncoderDevRef"=w519) -> ("Distance"=w517:dbl, "EncoderDevRef"=w511:T3)  [unwired: 5 in, 4 out]
        n153 = Greater?(x=w509, y=4.0) -> (0:w502:bool)
        n154 = Greater?(x=w517, y=4.0) -> (0:w503:bool)
        n155 = Select(t=0.0, s=w502, f=-0.3) -> (s? t:f=w505:dbl)
        n156 = Select(t=0.0, s=w503, f=-0.3) -> (s? t:f=w513:dbl)
        n157 = And(x=w503, y=w502) -> (x .and. y?=w501:bool)
        n158 = call <vilib>:"WPI_MotorControlSetOutput.vi"("Output"=w505, "MotorControlDevRef"=w504) -> ("MotorControlDevRef"=w499:T7)  [unwired: 7 in, 2 out]
        n159 = call <vilib>:"WPI_MotorControlSetOutput.vi"("Output"=w513, "MotorControlDevRef"=w518) -> ("MotorControlDevRef"=w512:T7)  [unwired: 7 in, 2 out]
      }
      n160 = while {
        tunnel: [w494] -> w421
        tunnel: [w493] -> w420
        tunnel: w429 -> [w492]
        tunnel: w428 -> [w491]
        tunnel: w423 -> [w487]
        tunnel: w422 -> [w486]
        tunnel: [w487] -> w419
        tunnel: [w486] -> w418
        tunnel: w412 -> [w485]
        tunnel: [w485] -> w411
        stop <- w488 continue-if-true
        n161 = call <vilib>:"WPI_EncoderGet.vi"("EncoderDevRef"=w492) -> ("Distance"=w490:dbl, "EncoderDevRef"=w494:T3)  [unwired: 5 in, 4 out]
        n162 = Greater?(x=4.0 ("y"), y=w490) -> (0:w488:bool)
        n163 = Select(t=0.3, s=w488, f=0.0 ("Output")) -> (s? t:f=w495:dbl)
        n164 = call <vilib>:"WPI_MotorControlSetOutput.vi"("Output"=w495, "MotorControlDevRef"=w491) -> ("MotorControlDevRef"=w493:T7)  [unwired: 7 in, 2 out]
      }
      n165 = while {
        tunnel: w421 -> [w484]
        tunnel: w420 -> [w483]
        tunnel: [w477] -> w414
        tunnel: [w476] -> w415
        tunnel: w419 -> [w475]
        tunnel: w418 -> [w469]
        tunnel: [w465] -> w416
        tunnel: [w464] -> w417
        tunnel: w411 -> [w463]
        tunnel: [w463] -> w410
        stop <- w466 stop-if-true
        n166 = call <vilib>:"WPI_EncoderGet.vi"("EncoderDevRef"=w475) -> ("Distance"=w474:dbl, "EncoderDevRef"=w465:T3)  [unwired: 5 in, 4 out]
        n167 = call <vilib>:"WPI_EncoderGet.vi"("EncoderDevRef"=w484) -> ("Distance"=w482:dbl, "EncoderDevRef"=w476:T3)  [unwired: 5 in, 4 out]
        n168 = Greater?(x=w474, y=4.0) -> (0:w467:bool)
        n169 = Greater?(x=w482, y=4.0) -> (0:w468:bool)
        n170 = Select(t=0.0, s=w467, f=-0.3) -> (s? t:f=w470:dbl)
        n171 = Select(t=0.0, s=w468, f=-0.3) -> (s? t:f=w478:dbl)
        n172 = And(x=w468, y=w467) -> (x .and. y?=w466:bool)
        n173 = call <vilib>:"WPI_MotorControlSetOutput.vi"("Output"=w470, "MotorControlDevRef"=w469) -> ("MotorControlDevRef"=w464:T7)  [unwired: 7 in, 2 out]
        n174 = call <vilib>:"WPI_MotorControlSetOutput.vi"("Output"=w478, "MotorControlDevRef"=w483) -> ("MotorControlDevRef"=w477:T7)  [unwired: 7 in, 2 out]
      }
      n175 = while {
        tunnel: w417 -> [w454]
        tunnel: w416 -> [w453]
        tunnel: w415 -> [w451]
        tunnel: w414 -> [w452]
        tunnel: w410 -> [w462]
        tunnel: [w454] -> w409
        tunnel: [w453] -> w408
        tunnel: [w452] -> w407
        tunnel: [w451] -> w406
        stop <- w455 stop-if-true
        n176 = global read "Robot Global Data.vi" "LOWER LIMIT"() -> (w458:bool)
        n177 = Select(t=0.0, s=w458, f=-0.5) -> (s? t:f=w459:dbl)
        n178 = call <vilib>:"WPI_MotorControlSetOutput.vi"("Output"=w459, "MotorControlDevRef"=w462) -> ("Motor Output"=w457:dbl)  [unwired: 7 in, 2 out]
        n179 = Equal?(x=w457, y=0.0) -> (x = y?=w455:bool)
      }
      n180 = while {
        tunnel: [w445] -> _
        tunnel: [w444] -> _
        tunnel: [w435] -> _
        tunnel: [w434] -> _
        tunnel: w409 -> [w433]
        tunnel: w408 -> [w432]
        tunnel: w407 -> [w431]
        tunnel: w406 -> [w430]
        stop <- w436 stop-if-true
        n181 = call <vilib>:"WPI_EncoderGet.vi"("EncoderDevRef"=w432) -> ("Distance"=w443:dbl, "EncoderDevRef"=w435:T3)  [unwired: 5 in, 4 out]
        n182 = call <vilib>:"WPI_EncoderGet.vi"("EncoderDevRef"=w430) -> ("Distance"=w450:dbl, "EncoderDevRef"=w444:T3)  [unwired: 5 in, 4 out]
        n183 = Greater?(x=w443, y=0.0) -> (0:w437:bool)
        n184 = Greater?(x=w450, y=0.0) -> (0:w438:bool)
        n185 = Select(t=-0.3, s=w437, f=0.0) -> (s? t:f=w439:dbl)
        n186 = Select(t=-0.3, s=w438, f=0.0) -> (s? t:f=w446:dbl)
        n187 = And(x=w438, y=w437) -> (x .and. y?=w436:bool)
        n188 = call <vilib>:"WPI_MotorControlSetOutput.vi"("Output"=w439, "MotorControlDevRef"=w433) -> ("MotorControlDevRef"=w434:T7)  [unwired: 7 in, 2 out]
        n189 = call <vilib>:"WPI_MotorControlSetOutput.vi"("Output"=w446, "MotorControlDevRef"=w431) -> ("MotorControlDevRef"=w445:T7)  [unwired: 7 in, 2 out]
      }
    }
    frame "GEAR1" {
      n190 = while {
        tunnel: w538 -> [w619]
        tunnel: w539 -> [w599]
        tunnel: [w615] -> w534
        tunnel: [w614] -> w529
        tunnel: w537 -> [w606]
        tunnel: w536 -> [w603]
        tunnel: [w606] -> w527
        tunnel: [w610] -> w533
        tunnel: w535 -> [w609]
        tunnel: [w609] -> w531
        stop <- w604 continue-if-true
        n191 = call <vilib>:"WPI_CANTalonSRX_GetStatus.vi"("CAN Talon SRX Ref"=w599) -> ("Talon SRX Status"=w597:T15, "CAN Talon SRX Ref"=w598:T7)  [unwired: 8 in, 1 out]
        n192 = call <vilib>:"WPI_CANTalonSRX_GetStatus.vi"("CAN Talon SRX Ref"=w603) -> ("Talon SRX Status"=w601:T15, "CAN Talon SRX Ref"=w602:T7)  [unwired: 8 in, 1 out]
        n193 = Unbundle By Name(w601) -> ("Current"=→"CURRENT":dbl)
        n194 = call <vilib>:"WPI_EncoderGet.vi"("EncoderDevRef"=w619) -> ("Distance"=w605:dbl, "EncoderDevRef"=w614:T3)  [unwired: 5 in, 4 out]
        "Distance" <- w605
        n195 = Unbundle By Name(w597) -> ("Current"=→"Current":dbl)
        n196 = In Range and Coerce(upper limit=15.9, x=w605, lower limit=0.0) -> (In Range?=w604:bool)  [unwired: 1 out]
        n197 = Select(t=0.3, s=w604, f=0.0) -> (s? t:f=w611:dbl)
        n198 = Select(t=0.3, s=w604, f=0.0) -> (s? t:f=w616:dbl)
        n199 = call <vilib>:"WPI_MotorControlSetOutput.vi"("Output"=w611, "MotorControlDevRef"=w602) -> ("MotorControlDevRef"=w610:T7)  [unwired: 7 in, 2 out]
        n200 = call <vilib>:"WPI_MotorControlSetOutput.vi"("Output"=w616, "MotorControlDevRef"=w598) -> ("MotorControlDevRef"=w615:T7)  [unwired: 7 in, 2 out]
      }
      n201 = call <vilib>:"WPI_EncoderReset.vi"("EncoderDevRef"=w529) -> ("EncoderDevRef"=w528:T3)  [unwired: 9 in, 1 out]
      n202 = while {
        tunnel: [w575] -> w532
        tunnel: [w574] -> w526
        tunnel: [w570] -> w523
        tunnel: w528 -> [w566]
        tunnel: w534 -> [w565]
        tunnel: w533 -> [w564]
        tunnel: [w563] -> w530
        tunnel: w531 -> [w563]
        tunnel: w527 -> [w562]
        stop <- w556 continue-if-true
        n203 = call <vilib>:"WPI_EncoderGet.vi"("EncoderDevRef"=w562) -> ("Distance"=w561:dbl)  [unwired: 5 in, 5 out]
        n204 = call <vilib>:"WPI_EncoderGet.vi"("EncoderDevRef"=w566) -> ("Distance"=w567:dbl, "EncoderDevRef"=w574:T3)  [unwired: 5 in, 4 out]
        n205 = In Range and Coerce(upper limit=0.4, x=w561, lower limit=0.0) -> (In Range?=w558:bool)  [unwired: 1 out]
        n206 = In Range and Coerce(upper limit=5.9, x=w567, lower limit=0.0) -> (In Range?=w557:bool)  [unwired: 1 out]
        n207 = Select(t=0.3, s=w558, f=0.0) -> (s? t:f=w571:dbl)
        n208 = Select(t=-0.3, s=w557, f=0.0) -> (s? t:f=w576:dbl)
        n209 = And(x=w558, y=w557) -> (x .and. y?=w556:bool)
        n210 = call <vilib>:"WPI_MotorControlSetOutput.vi"("Output"=w571, "MotorControlDevRef"=w564) -> ("MotorControlDevRef"=w570:T7)  [unwired: 7 in, 2 out]
        n211 = call <vilib>:"WPI_MotorControlSetOutput.vi"("Output"=w576, "MotorControlDevRef"=w565) -> ("MotorControlDevRef"=w575:T7)  [unwired: 7 in, 2 out]
      }
      n212 = call <vilib>:"WPI_EncoderReset.vi"("EncoderDevRef"=w526) -> ("EncoderDevRef"=w525:T3)  [unwired: 9 in, 1 out]
      n213 = while {
        tunnel: [w592] -> w522
        tunnel: [w591] -> w521
        tunnel: [w587] -> w520
        tunnel: w532 -> [w582]
        tunnel: w523 -> [w581]
        tunnel: w530 -> [w579]
        tunnel: w525 -> [w580]
        tunnel: [w579] -> _
        stop <- w583 continue-if-true
        n214 = call <vilib>:"WPI_EncoderGet.vi"("EncoderDevRef"=w580) -> ("Distance"=w584:dbl, "EncoderDevRef"=w591:T3)  [unwired: 5 in, 4 out]
        n215 = In Range and Coerce(upper limit=5.0, x=w584, lower limit=0.0) -> (In Range?=w583:bool)  [unwired: 1 out]
        n216 = Select(t=-0.3, s=w583, f=0.0) -> (s? t:f=w588:dbl)
        n217 = Select(t=-0.3, s=w583, f=0.0) -> (s? t:f=w593:dbl)
        n218 = call <vilib>:"WPI_MotorControlSetOutput.vi"("Output"=w588, "MotorControlDevRef"=w581) -> ("MotorControlDevRef"=w587:T7)  [unwired: 7 in, 2 out]
        n219 = call <vilib>:"WPI_MotorControlSetOutput.vi"("Output"=w593, "MotorControlDevRef"=w582) -> ("MotorControlDevRef"=w592:T7)  [unwired: 7 in, 2 out]
      }
      n220 = call <vilib>:"WPI_EncoderReset.vi"("EncoderDevRef"=w521) -> ("EncoderDevRef"=w524:T3)  [unwired: 9 in, 1 out]
      n221 = while {
        tunnel: [w552] -> _
        tunnel: [w551] -> _
        tunnel: [w547] -> _
        tunnel: w522 -> [w542]
        tunnel: w520 -> [w541]
        tunnel: w524 -> [w540]
        stop <- w543 continue-if-true
        n222 = call <vilib>:"WPI_EncoderGet.vi"("EncoderDevRef"=w540) -> ("Distance"=w544:dbl, "EncoderDevRef"=w551:T3)  [unwired: 5 in, 4 out]
        n223 = In Range and Coerce(upper limit=5.0, x=w544, lower limit=0.0) -> (In Range?=w543:bool)  [unwired: 1 out]
        n224 = Select(t=0.4, s=w543, f=0.0) -> (s? t:f=w548:dbl)
        n225 = Select(t=0.4, s=w543, f=0.0) -> (s? t:f=w553:dbl)
        n226 = call <vilib>:"WPI_MotorControlSetOutput.vi"("Output"=w548, "MotorControlDevRef"=w541) -> ("MotorControlDevRef"=w547:T7)  [unwired: 7 in, 2 out]
        n227 = call <vilib>:"WPI_MotorControlSetOutput.vi"("Output"=w553, "MotorControlDevRef"=w542) -> ("MotorControlDevRef"=w552:T7)  [unwired: 7 in, 2 out]
      }
    }
    frame "CENTERGEAR" {
      n228 = call-poly <vilib>:"WPI_RobotDriveArcadeDrive.vi"("error in (no error)"=w642, "Y axis value"=0.5, "RobotDriveDevRef"=w643) -> ("error out"=w639:errorcluster, "RobotDriveDevRef"=w640:T11)  [unwired: 6 in, 1 out]
      n229 = call <vilib>:"WPI_RobotDriveDelayAndUpdateSafety.vi"("error in (no error)"=w639, "Delay (s)"=3.0, "RobotDriveDevRef"=w640) -> ("error out"=w636:errorcluster, "RobotDriveDevRef 2"=w634:T11)  [unwired: 7 in]
      n230 = call <vilib>:"WPI_MotorControlSetOutput.vi"("error in (no error)"=w636, "Output"=-0.6, "MotorControlDevRef"=w637) -> ("error out"=w633:errorcluster)  [unwired: 6 in, 2 out]
      n231 = call <vilib>:"WPI_RobotDriveDelayAndUpdateSafety.vi"("error in (no error)"=w633, "Delay (s)"=2.0, "RobotDriveDevRef"=w634) -> ("error out"=w629:errorcluster, "RobotDriveDevRef 2"=w631:T11)  [unwired: 7 in]
      n232 = call-poly <vilib>:"WPI_RobotDriveArcadeDrive.vi"("error in (no error)"=w629, "Y axis value"=-0.4, "RobotDriveDevRef"=w631) -> ("error out"=w628:errorcluster, "RobotDriveDevRef"=w627:T11)  [unwired: 6 in, 1 out]
      n233 = call <vilib>:"WPI_RobotDriveDelayAndUpdateSafety.vi"("error in (no error)"=w628, "Delay (s)"=2.0, "RobotDriveDevRef"=w627) -> ("error out"=w624:errorcluster, "RobotDriveDevRef 2"=w625:T11)  [unwired: 7 in]
      n234 = call-poly <vilib>:"WPI_RobotDriveArcadeDrive.vi"("error in (no error)"=w624, "Y axis value"=0.0, "RobotDriveDevRef"=w625) -> ("error out"=w621:errorcluster, "RobotDriveDevRef"=w622:T11)  [unwired: 6 in, 1 out]
      n235 = call <vilib>:"WPI_RobotDriveDelayAndUpdateSafety.vi"("error in (no error)"=w621, "Delay (s)"=1.0, "RobotDriveDevRef"=w622) -> ()  [unwired: 7 in, 2 out]
    }
    frame "ENCODER" {
      n236 = while {
        tunnel: w657 -> [w712]
        tunnel: w656 -> [w710]
        tunnel: w655 -> [w711]
        tunnel: w654 -> [w709]
        tunnel: w653 -> [w691]
        tunnel: [w695] -> w652
        tunnel: [w694] -> w651
        tunnel: [w693] -> w650
        tunnel: [w692] -> w649
        tunnel: [w691] -> w648
        stop <- w696 continue-if-true
        n237 = call <vilib>:"WPI_EncoderGet.vi"("EncoderDevRef"=w711) -> ("Distance"=w702:dbl, "EncoderDevRef"=w692:T3)  [unwired: 5 in, 4 out]
        n238 = call <vilib>:"WPI_EncoderGet.vi"("EncoderDevRef"=w712) -> ("Distance"=w708:dbl, "EncoderDevRef"=w694:T3)  [unwired: 5 in, 4 out]
        n239 = Less?(x=w708, y=78.0) -> (x < y?=w698:bool)
        n240 = Less?(x=w702, y=78.0) -> (x < y?=w697:bool)
        n241 = Select(t=0.3, s=w698, f=0.0) -> (s? t:f=w704:dbl)
        n242 = Select(t=0.3, s=w697, f=0.0) -> (s? t:f=w700:dbl)
        n243 = And(x=w698, y=w697) -> (x .and. y?=w696:bool)
        n244 = call <vilib>:"WPI_MotorControlSetOutput.vi"("Output"=w704, "MotorControlDevRef"=w710) -> ("MotorControlDevRef"=w693:T7)  [unwired: 7 in, 2 out]
        n245 = call <vilib>:"WPI_MotorControlSetOutput.vi"("Output"=w700, "MotorControlDevRef"=w709) -> ("MotorControlDevRef"=w695:T7)  [unwired: 7 in, 2 out]
      }
      n246 = while {
        tunnel: w652 -> [w688]
        tunnel: w651 -> [w685]
        tunnel: w650 -> [w686]
        tunnel: w649 -> [w687]
        tunnel: w648 -> [w690]
        tunnel: [w688] -> w646
        tunnel: [w687] -> w644
        tunnel: [w686] -> w647
        tunnel: [w685] -> w645
        stop <- w684 stop-if-true
        n247 = Wait (ms)(milliseconds to wait=u32 3000) -> (millisecond timer value=w683:u32)
        n248 = call <vilib>:"WPI_MotorControlSetOutput.vi"("Output"=-0.6, "MotorControlDevRef"=w690) -> ()  [unwired: 7 in, 3 out]
        n249 = Equal?(x=w683, y=u32 3000) -> (x = y?=w684:bool)
      }
      n250 = flat-sequence {
        tunnel: w644 -> [w658]
        frame #0 {
          n251 = call <vilib>:"WPI_EncoderReset.vi"("EncoderDevRef"=w658) -> ()  [unwired: 9 in, 2 out]
        }
      }
      n252 = flat-sequence {
        tunnel: w645 -> [w659]
        frame #0 {
          n253 = call <vilib>:"WPI_EncoderReset.vi"("EncoderDevRef"=w659) -> ()  [unwired: 9 in, 2 out]
        }
      }
      n254 = while {
        tunnel: w645 -> [w680]
        tunnel: w647 -> [w679]
        tunnel: w646 -> [w678]
        tunnel: [w664] -> _
        tunnel: [w663] -> _
        tunnel: [w662] -> _
        tunnel: [w661] -> _
        tunnel: w644 -> [w660]
        stop <- w665 continue-if-true
        n255 = call <vilib>:"WPI_EncoderGet.vi"("EncoderDevRef"=w660) -> ("Distance"=w671:dbl, "EncoderDevRef"=w661:T3)  [unwired: 5 in, 4 out]
        n256 = call <vilib>:"WPI_EncoderGet.vi"("EncoderDevRef"=w680) -> ("Distance"=w677:dbl, "EncoderDevRef"=w663:T3)  [unwired: 5 in, 4 out]
        n257 = Less?(x=w677, y=-40.0) -> (x < y?=w667:bool)
        n258 = Less?(x=w671, y=-40.0) -> (x < y?=w666:bool)
        n259 = Select(t=-0.3, s=w667, f=0.0) -> (s? t:f=w673:dbl)
        n260 = Select(t=-0.3, s=w666, f=0.0) -> (s? t:f=w669:dbl)
        n261 = And(x=w667, y=w666) -> (x .and. y?=w665:bool)
        n262 = call <vilib>:"WPI_MotorControlSetOutput.vi"("Output"=w673, "MotorControlDevRef"=w679) -> ("MotorControlDevRef"=w662:T7)  [unwired: 7 in, 2 out]
        n263 = call <vilib>:"WPI_MotorControlSetOutput.vi"("Output"=w669, "MotorControlDevRef"=w678) -> ("MotorControlDevRef"=w664:T7)  [unwired: 7 in, 2 out]
      }
    }
    frame "AUTO CENTER" {
      n264 = while {
        tunnel: w726 -> [w781]
        tunnel: w725 -> [w780]
        tunnel: [w774] -> w717
        tunnel: [w773] -> w716
        tunnel: w724 -> [w772]
        tunnel: w723 -> [w766]
        tunnel: [w762] -> w715
        tunnel: [w761] -> w714
        tunnel: w722 -> [w760]
        tunnel: [w760] -> w713
        stop <- w763 stop-if-true
        n265 = call <vilib>:"WPI_EncoderGet.vi"("EncoderDevRef"=w772) -> ("Distance"=w771:dbl, "EncoderDevRef"=w762:T3)  [unwired: 5 in, 4 out]
        n266 = call <vilib>:"WPI_EncoderGet.vi"("EncoderDevRef"=w781) -> ("Distance"=w779:dbl, "EncoderDevRef"=w773:T3)  [unwired: 5 in, 4 out]
        n267 = Greater?(x=w771, y=4.0) -> (0:w764:bool)
        n268 = Greater?(x=w779, y=4.0) -> (0:w765:bool)
        n269 = Select(t=0.0, s=w764, f=-0.3) -> (s? t:f=w767:dbl)
        n270 = Select(t=0.0, s=w765, f=-0.3) -> (s? t:f=w775:dbl)
        n271 = And(x=w765, y=w764) -> (x .and. y?=w763:bool)
        n272 = call <vilib>:"WPI_MotorControlSetOutput.vi"("Output"=w767, "MotorControlDevRef"=w766) -> ("MotorControlDevRef"=w761:T7)  [unwired: 7 in, 2 out]
        n273 = call <vilib>:"WPI_MotorControlSetOutput.vi"("Output"=w775, "MotorControlDevRef"=w780) -> ("MotorControlDevRef"=w774:T7)  [unwired: 7 in, 2 out]
      }
      n274 = while {
        tunnel: w714 -> [w751]
        tunnel: w715 -> [w750]
        tunnel: w716 -> [w748]
        tunnel: w717 -> [w749]
        tunnel: w713 -> [w759]
        tunnel: [w751] -> w718
        tunnel: [w750] -> w719
        tunnel: [w749] -> w720
        tunnel: [w748] -> w721
        stop <- w752 stop-if-true
        n275 = global read "Robot Global Data.vi" "LOWER LIMIT"() -> (w755:bool)
        n276 = Select(t=0.0, s=w755, f=-0.5) -> (s? t:f=w756:dbl)
        n277 = call <vilib>:"WPI_MotorControlSetOutput.vi"("Output"=w756, "MotorControlDevRef"=w759) -> ("Motor Output"=w754:dbl)  [unwired: 7 in, 2 out]
        n278 = Equal?(x=w754, y=0.0) -> (x = y?=w752:bool)
      }
      n279 = while {
        tunnel: [w742] -> _
        tunnel: [w741] -> _
        tunnel: [w732] -> _
        tunnel: [w731] -> _
        tunnel: w718 -> [w730]
        tunnel: w719 -> [w729]
        tunnel: w720 -> [w728]
        tunnel: w721 -> [w727]
        stop <- w733 stop-if-true
        n280 = call <vilib>:"WPI_EncoderGet.vi"("EncoderDevRef"=w729) -> ("Distance"=w740:dbl, "EncoderDevRef"=w732:T3)  [unwired: 5 in, 4 out]
        n281 = call <vilib>:"WPI_EncoderGet.vi"("EncoderDevRef"=w727) -> ("Distance"=w747:dbl, "EncoderDevRef"=w741:T3)  [unwired: 5 in, 4 out]
        n282 = Greater?(x=w740, y=0.0) -> (0:w734:bool)
        n283 = Greater?(x=w747, y=0.0) -> (0:w735:bool)
        n284 = Select(t=-0.3, s=w734, f=0.0) -> (s? t:f=w736:dbl)
        n285 = Select(t=-0.3, s=w735, f=0.0) -> (s? t:f=w743:dbl)
        n286 = And(x=w735, y=w734) -> (x .and. y?=w733:bool)
        n287 = call <vilib>:"WPI_MotorControlSetOutput.vi"("Output"=w736, "MotorControlDevRef"=w730) -> ("MotorControlDevRef"=w731:T7)  [unwired: 7 in, 2 out]
        n288 = call <vilib>:"WPI_MotorControlSetOutput.vi"("Output"=w743, "MotorControlDevRef"=w728) -> ("MotorControlDevRef"=w742:T7)  [unwired: 7 in, 2 out]
      }
    }
    frame "AUTO LEFT NS" {
      n289 = while {
        tunnel: w802 -> [w859]
        tunnel: [w855] -> w799
        tunnel: [w854] -> w784
        tunnel: w801 -> [w850]
        tunnel: [w849] -> w798
        tunnel: w800 -> [w848]
        tunnel: [w848] -> w797
        tunnel: w782 -> [w843]
        stop <- w844 continue-if-true
        n290 = call <vilib>:"WPI_EncoderGet.vi"("EncoderDevRef"=w843) -> ("Distance"=w845:dbl, "EncoderDevRef"=w854:T3)  [unwired: 5 in, 4 out]
        "Distance 3" <- w845
        n291 = In Range and Coerce(upper limit=12.0, x=w845, lower limit=0.0) -> (In Range?=w844:bool)  [unwired: 1 out]
        n292 = Select(t=0.35, s=w844, f=0.0) -> (s? t:f=w851:dbl)
        n293 = Select(t=0.35, s=w844, f=0.0) -> (s? t:f=w856:dbl)
        n294 = call <vilib>:"WPI_MotorControlSetOutput.vi"("Output"=w851, "MotorControlDevRef"=w850) -> ("MotorControlDevRef"=w849:T7)  [unwired: 7 in, 2 out]
        n295 = call <vilib>:"WPI_MotorControlSetOutput.vi"("Output"=w856, "MotorControlDevRef"=w859) -> ("MotorControlDevRef"=w855:T7)  [unwired: 7 in, 2 out]
      }
      n296 = while {
        tunnel: w784 -> [w842]
        tunnel: w799 -> [w841]
        tunnel: [w837] -> w796
        tunnel: [w836] -> w783
        tunnel: w798 -> [w832]
        tunnel: [w831] -> w795
        tunnel: w797 -> [w830]
        tunnel: [w830] -> w794
        stop <- w826 continue-if-true
        n297 = call <vilib>:"WPI_EncoderGet.vi"("EncoderDevRef"=w842) -> ("Distance"=w827:dbl, "EncoderDevRef"=w836:T3)  [unwired: 5 in, 4 out]
        "Distance 4" <- w827
        n298 = In Range and Coerce(upper limit=2.4, x=w827, lower limit=0.0) -> (In Range?=w826:bool)  [unwired: 1 out]
        n299 = Select(t=0.0, s=w826, f=0.0) -> (s? t:f=w833:dbl)
        n300 = Select(t=0.35, s=w826, f=0.0) -> (s? t:f=w838:dbl)
        n301 = call <vilib>:"WPI_MotorControlSetOutput.vi"("Output"=w833, "MotorControlDevRef"=w832) -> ("MotorControlDevRef"=w831:T7)  [unwired: 7 in, 2 out]
        n302 = call <vilib>:"WPI_MotorControlSetOutput.vi"("Output"=w838, "MotorControlDevRef"=w841) -> ("MotorControlDevRef"=w837:T7)  [unwired: 7 in, 2 out]
      }
      n303 = flat-sequence {
        tunnel: w784 -> [w804]
        frame #0 {
          n304 = call <vilib>:"WPI_EncoderReset.vi"("EncoderDevRef"=w804) -> ()  [unwired: 9 in, 2 out]
        }
      }
      n305 = while {
        tunnel: w783 -> [w825]
        tunnel: w796 -> [w824]
        tunnel: [w820] -> w793
        tunnel: [w819] -> w792
        tunnel: w795 -> [w815]
        tunnel: [w814] -> w791
        tunnel: w794 -> [w813]
        tunnel: [w813] -> w790
        stop <- w809 continue-if-true
        n306 = call <vilib>:"WPI_EncoderGet.vi"("EncoderDevRef"=w825) -> ("Distance"=w810:dbl, "EncoderDevRef"=w819:T3)  [unwired: 5 in, 4 out]
        "Distance 5" <- w810
        n307 = In Range and Coerce(upper limit=4.0, x=w810, lower limit=0.0) -> (In Range?=w809:bool)  [unwired: 1 out]
        n308 = Select(t=0.35, s=w809, f=0.0) -> (s? t:f=w816:dbl)
        n309 = Select(t=0.35, s=w809, f=0.0) -> (s? t:f=w821:dbl)
        n310 = call <vilib>:"WPI_MotorControlSetOutput.vi"("Output"=w816, "MotorControlDevRef"=w815) -> ("MotorControlDevRef"=w814:T7)  [unwired: 7 in, 2 out]
        n311 = call <vilib>:"WPI_MotorControlSetOutput.vi"("Output"=w821, "MotorControlDevRef"=w824) -> ("MotorControlDevRef"=w820:T7)  [unwired: 7 in, 2 out]
      }
      n312 = flat-sequence {
        tunnel: w783 -> [w803]
        frame #0 {
          n313 = call <vilib>:"WPI_EncoderReset.vi"("EncoderDevRef"=w803) -> ()  [unwired: 9 in, 2 out]
        }
      }
      n314 = while {
        tunnel: w791 -> [w866]
        tunnel: w792 -> [w864]
        tunnel: w793 -> [w865]
        tunnel: w790 -> [w867]
        tunnel: [w866] -> w787
        tunnel: [w865] -> w789
        tunnel: [w864] -> w788
        tunnel: [w863] -> w786
        tunnel: [w860] -> w785
        stop <- w862 stop-if-true
        n315 = call <vilib>:"WPI_MotorControlSetOutput.vi"("Output"=-0.5 ("f"), "MotorControlDevRef"=w867) -> ("error out"=w860:errorcluster, "MotorControlDevRef"=w863:T7)  [unwired: 7 in, 1 out]
        n316 = global read "Robot Global Data.vi" "LOWER LIMIT"() -> (w862:bool)
      }
      n317 = while {
        tunnel: w789 -> [_]
        tunnel: w788 -> [_]
        tunnel: w787 -> [_]
        tunnel: w786 -> [w807]
        tunnel: w785 -> [w806]
        stop <- FALSE stop-if-true
        n318 = call <vilib>:"WPI_MotorControlSetOutput.vi"("error in (no error)"=w806, "Output"=0.0, "MotorControlDevRef"=w807) -> ()  [unwired: 6 in, 3 out]
      }
    }
    frame "MIDDLE" {
      n319 = call-poly <vilib>:"WPI_RobotDriveArcadeDrive.vi"("error in (no error)"=w897, "Y axis value"=0.45, "RobotDriveDevRef"=w898) -> ("error out"=w894:errorcluster, "RobotDriveDevRef"=w895:T11)  [unwired: 6 in, 1 out]
      n320 = call <vilib>:"WPI_RobotDriveDelayAndUpdateSafety.vi"("error in (no error)"=w894, "Delay (s)"=2.0, "RobotDriveDevRef"=w895) -> ("error out"=w892:errorcluster, "RobotDriveDevRef 2"=w891:T11)  [unwired: 7 in]
      n321 = call-poly <vilib>:"WPI_RobotDriveArcadeDrive.vi"("error in (no error)"=w892, "Y axis value"=0.0, "RobotDriveDevRef"=w891) -> ("error out"=w888:errorcluster, "RobotDriveDevRef"=w889:T11)  [unwired: 6 in, 1 out]
      n322 = call <vilib>:"WPI_RobotDriveDelayAndUpdateSafety.vi"("error in (no error)"=w888, "Delay (s)"=0.5, "RobotDriveDevRef"=w889) -> ("error out"=w886:errorcluster, "RobotDriveDevRef 2"=w884:T11)  [unwired: 7 in]
      n323 = call <vilib>:"WPI_MotorControlSetOutput.vi"("error in (no error)"=w886, "Output"=-0.7, "MotorControlDevRef"=w885) -> ("error out"=w883:errorcluster, "MotorControlDevRef"=w879:T7)  [unwired: 6 in, 1 out]
      n324 = call <vilib>:"WPI_RobotDriveDelayAndUpdateSafety.vi"("error in (no error)"=w883, "Delay (s)"=1.5, "RobotDriveDevRef"=w884) -> ("error out"=w880:errorcluster, "RobotDriveDevRef 2"=w877:T11)  [unwired: 7 in]
      n325 = call <vilib>:"WPI_MotorControlSetOutput.vi"("error in (no error)"=w880, "Output"=0.0, "MotorControlDevRef"=w879) -> ("error out"=w876:errorcluster)  [unwired: 6 in, 2 out]
      n326 = call-poly <vilib>:"WPI_RobotDriveArcadeDrive.vi"("error in (no error)"=w876, "Y axis value"=-0.4, "RobotDriveDevRef"=w877) -> ("error out"=w873:errorcluster, "RobotDriveDevRef"=w874:T11)  [unwired: 6 in, 1 out]
      n327 = call <vilib>:"WPI_RobotDriveDelayAndUpdateSafety.vi"("error in (no error)"=w873, "Delay (s)"=2.0, "RobotDriveDevRef"=w874) -> ("error out"=w870:errorcluster, "RobotDriveDevRef 2"=w871:T11)  [unwired: 7 in]
      n328 = call-poly <vilib>:"WPI_RobotDriveArcadeDrive.vi"("error in (no error)"=w870, "Y axis value"=0.0, "X axis value"=0.0, "RobotDriveDevRef"=w871) -> ()  [unwired: 5 in, 3 out]
    }
    frame "RIGHTSIDE" {
      # "RIGHTSIDE"
      n329 = call-poly <vilib>:"WPI_RobotDriveArcadeDrive.vi"("error in (no error)"=w900, "Y axis value"=0.59, "RobotDriveDevRef"=w901) -> ("error out"=w940:errorcluster, "RobotDriveDevRef"=w941:T11)  [unwired: 6 in, 1 out]
      n330 = call <vilib>:"WPI_RobotDriveDelayAndUpdateSafety.vi"("error in (no error)"=w940, "Delay (s)"=1.8, "RobotDriveDevRef"=w941) -> ("error out"=w936:errorcluster, "RobotDriveDevRef 2"=w937:T11)  [unwired: 7 in]
      n331 = call-poly <vilib>:"WPI_RobotDriveArcadeDrive.vi"("error in (no error)"=w936, "X axis value"=0.36, "RobotDriveDevRef"=w937) -> ("error out"=w933:errorcluster, "RobotDriveDevRef"=w934:T11)  [unwired: 6 in, 1 out]
      n332 = call <vilib>:"WPI_RobotDriveDelayAndUpdateSafety.vi"("error in (no error)"=w933, "Delay (s)"=1.0, "RobotDriveDevRef"=w934) -> ("error out"=w930:errorcluster, "RobotDriveDevRef 2"=w931:T11)  [unwired: 7 in]
      n333 = call-poly <vilib>:"WPI_RobotDriveArcadeDrive.vi"("error in (no error)"=w930, "Y axis value"=0.5, "RobotDriveDevRef"=w931) -> ("error out"=w927:errorcluster, "RobotDriveDevRef"=w928:T11)  [unwired: 6 in, 1 out]
      n334 = call <vilib>:"WPI_RobotDriveDelayAndUpdateSafety.vi"("error in (no error)"=w927, "Delay (s)"=2.3, "RobotDriveDevRef"=w928) -> ("error out"=w924:errorcluster, "RobotDriveDevRef 2"=w925:T11)  [unwired: 7 in]
      n335 = call-poly <vilib>:"WPI_RobotDriveArcadeDrive.vi"("error in (no error)"=w924, "Y axis value"=0.0, "RobotDriveDevRef"=w925) -> ("error out"=w921:errorcluster, "RobotDriveDevRef"=w922:T11)  [unwired: 6 in, 1 out]
      n336 = call <vilib>:"WPI_RobotDriveDelayAndUpdateSafety.vi"("error in (no error)"=w921, "Delay (s)"=0.5, "RobotDriveDevRef"=w922) -> ("error out"=w919:errorcluster, "RobotDriveDevRef 2"=w917:T11)  [unwired: 7 in]
      n337 = call <vilib>:"WPI_MotorControlSetOutput.vi"("error in (no error)"=w919, "Output"=-0.7, "MotorControlDevRef"=w899) -> ("error out"=w916:errorcluster, "MotorControlDevRef"=w905:T7)  [unwired: 6 in, 1 out]
      n338 = call <vilib>:"WPI_RobotDriveDelayAndUpdateSafety.vi"("error in (no error)"=w916, "Delay (s)"=1.5, "RobotDriveDevRef"=w917) -> ("error out"=w904:errorcluster, "RobotDriveDevRef 2"=w914:T11)  [unwired: 7 in]
      n339 = call <vilib>:"WPI_MotorControlSetOutput.vi"("error in (no error)"=w904, "Output"=0.0, "MotorControlDevRef"=w905) -> ("error out"=w902:errorcluster)  [unwired: 6 in, 2 out]
      n340 = call-poly <vilib>:"WPI_RobotDriveArcadeDrive.vi"("error in (no error)"=w902, "Y axis value"=-0.4, "RobotDriveDevRef"=w914) -> ("error out"=w911:errorcluster, "RobotDriveDevRef"=w912:T11)  [unwired: 6 in, 1 out]
      n341 = call <vilib>:"WPI_RobotDriveDelayAndUpdateSafety.vi"("error in (no error)"=w911, "Delay (s)"=2.0, "RobotDriveDevRef"=w912) -> ("error out"=w909:errorcluster, "RobotDriveDevRef 2"=w908:T11)  [unwired: 7 in]
      n342 = call-poly <vilib>:"WPI_RobotDriveArcadeDrive.vi"("error in (no error)"=w909, "Y axis value"=0.0, "X axis value"=0.0, "RobotDriveDevRef"=w908) -> ()  [unwired: 5 in, 3 out]
    }
    frame "LEFTSIDE" {
      n343 = call-poly <vilib>:"WPI_RobotDriveArcadeDrive.vi"("error in (no error)"=w983, "Y axis value"=0.6, "RobotDriveDevRef"=w984) -> ("error out"=w981:errorcluster, "RobotDriveDevRef"=w982:T11)  [unwired: 6 in, 1 out]
      n344 = call <vilib>:"WPI_RobotDriveDelayAndUpdateSafety.vi"("error in (no error)"=w981, "Delay (s)"=2.0, "RobotDriveDevRef"=w982) -> ("error out"=w977:errorcluster, "RobotDriveDevRef 2"=w978:T11)  [unwired: 7 in]
      n345 = call-poly <vilib>:"WPI_RobotDriveArcadeDrive.vi"("error in (no error)"=w977, "X axis value"=-0.45, "RobotDriveDevRef"=w978) -> ("error out"=w974:errorcluster, "RobotDriveDevRef"=w975:T11)  [unwired: 6 in, 1 out]
      n346 = call <vilib>:"WPI_RobotDriveDelayAndUpdateSafety.vi"("error in (no error)"=w974, "Delay (s)"=1.0, "RobotDriveDevRef"=w975) -> ("error out"=w971:errorcluster, "RobotDriveDevRef 2"=w972:T11)  [unwired: 7 in]
      n347 = call-poly <vilib>:"WPI_RobotDriveArcadeDrive.vi"("error in (no error)"=w971, "Y axis value"=0.52, "RobotDriveDevRef"=w972) -> ("error out"=w968:errorcluster, "RobotDriveDevRef"=w969:T11)  [unwired: 6 in, 1 out]
      n348 = call <vilib>:"WPI_RobotDriveDelayAndUpdateSafety.vi"("error in (no error)"=w968, "Delay (s)"=2.25, "RobotDriveDevRef"=w969) -> ("error out"=w965:errorcluster, "RobotDriveDevRef 2"=w966:T11)  [unwired: 7 in]
      n349 = call-poly <vilib>:"WPI_RobotDriveArcadeDrive.vi"("error in (no error)"=w965, "Y axis value"=0.0, "RobotDriveDevRef"=w966) -> ("error out"=w962:errorcluster, "RobotDriveDevRef"=w963:T11)  [unwired: 6 in, 1 out]
      n350 = call <vilib>:"WPI_RobotDriveDelayAndUpdateSafety.vi"("error in (no error)"=w962, "Delay (s)"=0.5, "RobotDriveDevRef"=w963) -> ("error out"=w959:errorcluster, "RobotDriveDevRef 2"=w957:T11)  [unwired: 7 in]
      n351 = call <vilib>:"WPI_MotorControlSetOutput.vi"("error in (no error)"=w959, "Output"=-0.7, "MotorControlDevRef"=w960) -> ("error out"=w956:errorcluster, "MotorControlDevRef"=w945:T7)  [unwired: 6 in, 1 out]
      n352 = call <vilib>:"WPI_RobotDriveDelayAndUpdateSafety.vi"("error in (no error)"=w956, "Delay (s)"=1.5, "RobotDriveDevRef"=w957) -> ("error out"=w944:errorcluster, "RobotDriveDevRef 2"=w954:T11)  [unwired: 7 in]
      n353 = call <vilib>:"WPI_MotorControlSetOutput.vi"("error in (no error)"=w944, "Output"=0.0, "MotorControlDevRef"=w945) -> ("error out"=w942:errorcluster)  [unwired: 6 in, 2 out]
      n354 = call-poly <vilib>:"WPI_RobotDriveArcadeDrive.vi"("error in (no error)"=w942, "Y axis value"=-0.4, "RobotDriveDevRef"=w954) -> ("error out"=w951:errorcluster, "RobotDriveDevRef"=w952:T11)  [unwired: 6 in, 1 out]
      n355 = call <vilib>:"WPI_RobotDriveDelayAndUpdateSafety.vi"("error in (no error)"=w951, "Delay (s)"=2.0, "RobotDriveDevRef"=w952) -> ("error out"=w949:errorcluster, "RobotDriveDevRef 2"=w948:T11)  [unwired: 7 in]
      n356 = call-poly <vilib>:"WPI_RobotDriveArcadeDrive.vi"("error in (no error)"=w949, "Y axis value"=0.0, "X axis value"=0.0, "RobotDriveDevRef"=w948) -> ()  [unwired: 5 in, 3 out]
    }
    frame "Forward" {
      n357 = call-poly <vilib>:"WPI_RobotDriveArcadeDrive.vi"("error in (no error)"=w989, "Y axis value"=0.55, "RobotDriveDevRef"=w990) -> ("error out"=w985:errorcluster, "RobotDriveDevRef"=w987:T11)  [unwired: 6 in, 1 out]
      n358 = call <vilib>:"WPI_RobotDriveDelayAndUpdateSafety.vi"("error in (no error)"=w985, "Delay (s)"=2.8, "RobotDriveDevRef"=w987) -> ()  [unwired: 7 in, 2 out]
    }
    frame "GEAR DROP" {
      n359 = call-poly <vilib>:"WPI_RobotDriveArcadeDrive.vi"("error in (no error)"=w1014, "Y axis value"=0.45, "RobotDriveDevRef"=w1015) -> ("error out"=w1011:errorcluster, "RobotDriveDevRef"=w1012:T11)  [unwired: 6 in, 1 out]
      n360 = call <vilib>:"WPI_RobotDriveDelayAndUpdateSafety.vi"("error in (no error)"=w1011, "Delay (s)"=2.4, "RobotDriveDevRef"=w1012) -> ("error out"=w1009:errorcluster, "RobotDriveDevRef 2"=w1008:T11)  [unwired: 7 in]
      n361 = call-poly <vilib>:"WPI_RobotDriveArcadeDrive.vi"("error in (no error)"=w1009, "Y axis value"=0.0, "RobotDriveDevRef"=w1008) -> ("error out"=w1005:errorcluster, "RobotDriveDevRef"=w1006:T11)  [unwired: 6 in, 1 out]
      n362 = call <vilib>:"WPI_RobotDriveDelayAndUpdateSafety.vi"("error in (no error)"=w1005, "Delay (s)"=0.5, "RobotDriveDevRef"=w1006) -> ("error out"=w998:errorcluster, "RobotDriveDevRef 2"=w997:T11)  [unwired: 7 in]
      n363 = while {
        tunnel: w998 -> [w1027]
        tunnel: [w1024] -> w996
        tunnel: w995 -> [w1023]
        tunnel: [w1022] -> w994
        stop <- w1025 stop-if-true
        n364 = global read "Robot Global Data.vi" "LOWER LIMIT"() -> (w1025:bool)
        n365 = call <vilib>:"WPI_MotorControlSetOutput.vi"("error in (no error)"=w1027, "Output"=-0.6 ("f"), "MotorControlDevRef"=w1023) -> ("error out"=w1024:errorcluster, "MotorControlDevRef"=w1022:T7)  [unwired: 6 in, 1 out]
      }
      n366 = call-poly <vilib>:"WPI_RobotDriveArcadeDrive.vi"("error in (no error)"=w996, "Y axis value"=-0.4, "RobotDriveDevRef"=w997) -> ("error out"=w1002:errorcluster, "RobotDriveDevRef"=w1001:T11)  [unwired: 6 in, 1 out]
      n367 = call <vilib>:"WPI_RobotDriveDelayAndUpdateSafety.vi"("error in (no error)"=w1002, "Delay (s)"=1.5, "RobotDriveDevRef"=w1001) -> ("error out"=w993:errorcluster)  [unwired: 7 in, 1 out]
      n368 = while {
        tunnel: w994 -> [w1020]
        tunnel: w993 -> [w1018]
        tunnel: [w1017] -> w992
        tunnel: [w1016] -> w991
        stop <- w1021 stop-if-true
        n369 = call <vilib>:"WPI_MotorControlSetOutput.vi"("error in (no error)"=w1018, "Output"=0.6, "MotorControlDevRef"=w1020) -> ("error out"=w1016:errorcluster, "MotorControlDevRef"=w1017:T7)  [unwired: 6 in, 1 out]
        n370 = global read "Robot Global Data.vi" "UPPER LIMIT"() -> (w1021:bool)
      }
      n371 = call <vilib>:"WPI_MotorControlSetOutput.vi"("error in (no error)"=w991, "Output"=0.0, "MotorControlDevRef"=w992) -> ()  [unwired: 6 in, 3 out]
    }
  }
